vi "Telemetry Display.vi"() -> ()   [LabVIEW 2015]
uses:
  FPGA Telemetry.ctl
  Vehicle Status/Subsystem Status.ctl
  Vehicle Status/Subsystem Status Severity.ctl
  Vehicle Status/Subsystem Status Message.ctl
  AIR Status.ctl
  Reason for Shutdown.ctl
  Dash LED Status.ctl
  FPGA/SPI v2/ADXL345 Output.ctl
  CAN/MC/MC Telemetry.ctl
  CAN/MC/MC Temp 1.ctl
  CAN/MC/MC Temp 2.ctl
  CAN/MC/MC Temp 3.ctl
  CAN/MC/MC Current.ctl
  CAN/MC/MC Voltage.ctl
  CAN/MC/MC State.ctl
  CAN/Inverter States.ctl
  CAN/Inverter Run Modes.ctl
  CAN/VSM States.ctl
  CAN/MC/MC Torque.ctl
  CAN/MC/MC Position.ctl
  CAN/MC/MC Faults.ctl
  CAN/MC/MC Flux.ctl
  CAN/MC/MC Internal Voltages.ctl
  CAN/MC/MC Mod Index and Flux Weakening.ctl
  BMS Telemetry.ctl
  Session Information.ctl
  <vilib>/Math Plots/3D Math Plots/3D Bar/3D Bar XCtrl/3D Bar.xctl
  <vilib>/Math Plots/3D Math Plots/3D Bar/3D Bar Datatype/3D Bar Datatype.lvclass
  Vehicle Status/Remote Stop Type.ctl
  <vilib>/Math Plots/3D Math Plots/3D Bar/3D Bar Datatype/Public/Plot Helper (Matrix).vi
panel:
  out "Cell Temps":refnum<class "3D Plot Datatype.lvclass">[](xcontrol)
  out "Cell Voltages":refnum<class "3D Plot Datatype.lvclass">[](xcontrol)
  out "Waveform Chart":dbl(graph)=1.6
  out "Session Information":T1={"CLogFilePrefix"="110616 214028", "CExtraNotes"="", "CCircuit"="", "CCarName"="", "CDriverName"="", "CSessionDescription"=""}
  in  "Transmit":bool=TRUE
  in  "New TDMS Files":bool
  out "BMS Telemetry":T2={"bBMSIgnition"=FALSE, "bBMSChargerMains"=FALSE, "bBMSFastCharge"=FALSE, "bBMSChargerEnabled"=FALSE, "eBMSCarState"=enum."Off", "eBMSChargingState"=enum."Main Charging", "tBMSChargeStage"=12, "eBMSLastChargeError"=enum."No Error", "NBMSNumCells"=70, "bBMSUnderVProtection"=FALSE, "bBMSOverVProtection"=FALSE, "bBMSOverTProtection"=FALSE, "bBMSLeakageProtection"=FALSE, "bBMSNoCellCommsError"=FALSE, "bBMSLowVReduction"=FALSE, "bBMSHighTReduction"=FALSE, "VCellMin"=3.87, "VCellMax"=3.92, "VCellMean"=3.9, "VTotal"=273.18, "TCellMin"=29.0, "TCellMax"=42.0, "TCellMean"=32.0, "VCells"={"[0]"=3.91, "[1]"=3.9, "[2]"=3.9, "[3]"=3.9, "[4]"=3.91, "[5]"=3.91, "[6]"=3.91, "[7]"=3.9, "[8]"=3.92, "[9]"=3.9, "[10]"=3.91, "[11]"=3.9, "[12]"=3.9, "[13]"=3.9, "[14]"=3.9, "[15]"=3.9, "[16]"=3.92, "[16] 2"=0.0, "[17]"=3.9, "[18]"=3.91, "[19]"=3.9, "[20]"=3.91, "[21]"=3.9, "[22]"=3.9, "[23]"=3.91, "[24]"=3.91, "[25]"=3.91, "[26]"=3.9, "[27]"=3.9, "[28]"=3.9, "[29]"=3.9, "[30]"=3.9, "[31]"=3.9, "[32]"=3.9, "[33]"=3.91, "[33] 2"=0.0, "[34]"=3.91, "[35]"=3.91, "[36]"=3.9, "[37]"=3.9, "[38]"=3.91, "[39]"=3.91, "[40]"=3.91, "[41]"=3.9, "[42]"=3.9, "[43]"=3.91, "[44]"=3.9, "[45]"=3.8899999999999997, "[46]"=3.91, "[47]"=3.9, "[48]"=3.9, "[49]"=3.9, "[50]"=3.9, "[50] 2"=0.0, "[51]"=3.91, "[52] 2"=3.91, "[54]"=3.9, "[53]"=3.9, "[55]"=3.9, "[56]"=3.9, "[57]"=3.91, "[58]"=3.9, "[59]"=3.9, "[60]"=3.9, "[61]"=3.91, "[62]"=3.87, "[63]"=3.9, "[64]"=3.9, "[65]"=3.9, "[66]"=3.9, "[67]"=3.91}, "TBMSCells"={"[55]"=32.0, "[56]"=32.0, "[57]"=32.0, "[58]"=34.0, "[59]"=33.0, "[60]"=34.0, "[61]"=33.0, "[62]"=32.0, "[63]"=36.0, "[64]"=36.0, "[65]"=32.0, "[66]"=33.0, "[67]"=34.0, "[68]"=32.0, "[69]"=30.0, "[70]"=31.0, "[17]"=30.0, "[38]"=30.0, "[39]"=29.0, "[40]"=30.0, "[41]"=29.0, "[42]"=30.0, "[43]"=31.0, "[44]"=30.0, "[45]"=30.0, "[46]"=30.0, "[47]"=31.0, "[48]"=30.0, "[49]"=32.0, "[50]"=32.0, "[51]"=31.0, "[52]"=32.0, "[53]"=32.0, "[54]"=32.0, "[21]"=32.0, "[22]"=32.0, "[23]"=32.0, "[24]"=34.0, "[25]"=32.0, "[26]"=34.0, "[27]"=36.0, "[28]"=36.0, "[29]"=32.0, "[30]"=32.0, "[31]"=32.0, "[32]"=32.0, "[33]"=30.0, "[34]"=31.0, "[35]"=33.0, "[36]"=33.0, "[37]"=31.0, "[0]"=32.0, "[1]"=31.0, "[2]"=31.0, "[3]"=31.0, "[4]"=32.0, "[5]"=42.0, "[6]"=42.0, "[7]"=32.0, "[8]"=36.0, "[9]"=32.0, "[10]"=38.0, "[11]"=33.0, "[12]"=37.0, "[13]"=34.0, "[14]"=34.0, "[15]"=33.0, "[16]"=37.0}, "bChargerConnected"=TRUE, "VChargerSetpoint"=298.90000000000003, "IChargerSetpoint"=6.0, "VChargerActual"=277.7, "IChargerActual"=4.800000000000001, "BCells"={"[51]"=0.0, "[52]"=0.0, "[53]"=0.0, "[54]"=0.0, "[55]"=0.0, "[56]"=0.0, "[57]"=0.7843137254901961, "[58]"=0.0, "[59]"=1.5686274509803921, "[60]"=1.5686274509803921, "[61]"=0.0, "[62]"=0.0, "[63]"=0.7843137254901961, "[64]"=0.0, "[65]"=0.0, "[66]"=0.0, "[67]"=0.39215686274509803, "[34]"=0.39215686274509803, "[35]"=0.0, "[36]"=0.0, "[37]"=0.0, "[38]"=0.0, "[39]"=0.7843137254901961, "[40]"=0.0, "[41]"=0.0, "[42]"=0.0, "[43]"=8.627450980392156, "[44]"=0.0, "[45]"=0.0, "[46]"=0.7843137254901961, "[47]"=0.0, "[48]"=0.0, "[49]"=0.0, "[50]"=0.0, "[17]"=0.0, "[18]"=2.3529411764705883, "[19]"=0.0, "[20]"=0.0, "[21]"=0.0, "[22]"=0.0, "[23]"=1.5686274509803921, "[24]"=1.5686274509803921, "[25]"=0.0, "[26]"=0.0, "[27]"=0.0, "[28]"=0.0, "[29]"=0.0, "[30]"=0.0, "[31]"=0.0, "[32]"=0.0, "[33]"=0.0, "[0]"=0.0, "[1]"=0.0, "[2]"=0.0, "[3]"=0.0, "[4]"=1.9607843137254901, "[5]"=32.15686274509804, "[6]"=32.15686274509804, "[7]"=0.0, "[8]"=1.5686274509803921, "[9]"=0.0, "[10]"=16.07843137254902, "[11]"=0.0, "[12]"=3.9215686274509802, "[13]"=0.0, "[14]"=0.0, "[15]"=0.0, "[16]"=0.7843137254901961}, "bNewVCellMinSample"=TRUE, "Battery Temp"={"[0]"=0.0, "[1]"=0.0, "[2]"=0.0, "[3]"=0.0, "[4]"=0.0, "[5]"=0.0, "[6]"=0.0, "[7]"=0.0, "[8]"=0.0, "[9]"=0.0, "[10]"=0.0, "[11]"=0.0, "[12]"=0.0, "[13]"=0.0, "[14]"=0.0, "[15]"=0.0, "[16]"=0.0, "[17]"=0.0, "[18]"=0.0, "[19]"=0.0, "[20]"=0.0, "[21]"=0.0, "[22]"=0.0, "[23]"=0.0, "[24]"=0.0, "[25]"=0.0, "[26]"=0.0, "[27]"=0.0, "[28]"=0.0, "[29]"=0.0, "[30]"=0.0, "[31]"=0.0, "[32]"=0.0, "[33]"=0.0, "[34]"=0.0, "[35]"=0.0, "[36]"=0.0, "[37]"=0.0, "[38]"=0.0, "[39]"=0.0, "[40]"=0.0, "[41]"=0.0, "[42]"=0.0, "[43]"=0.0, "[44]"=0.0, "[45]"=0.0, "[46]"=0.0, "[47]"=0.0, "[48]"=0.0, "[49]"=0.0, "[50]"=0.0, "[51]"=0.0, "[52]"=0.0, "[53]"=0.0, "[54]"=0.0, "[55]"=0.0, "[56]"=0.0, "[57]"=0.0, "[58]"=0.0, "[59]"=0.0, "[60]"=0.0, "[61]"=0.0, "[62]"=0.0, "[63]"=0.0, "[64]"=0.0, "[65]"=0.0, "[66]"=0.0, "[67]"=0.0, "[68]"=0.0, "[69]"=0.0, "[71]"=0.0, "[70]"=0.0, "[0] 2"=0.0, "[1] 2"=0.0, "[2] 2"=0.0, "[3] 2"=0.0, "[4] 2"=0.0, "[5] 2"=0.0, "[6] 2"=0.0, "[7] 2"=0.0, "[8] 2"=0.0, "[9] 2"=0.0, "[10] 2"=0.0, "[11] 2"=0.0, "[12] 2"=0.0, "[13] 2"=0.0, "[14] 2"=0.0, "[15] 2"=0.0, "[16] 2"=0.0, "[17] 2"=0.0, "[18] 2"=0.0, "[19] 2"=0.0, "[20] 2"=0.0, "[21] 2"=0.0, "[22] 2"=0.0, "[23] 2"=0.0, "[24] 2"=0.0, "[25] 2"=0.0, "[26] 2"=0.0, "[27] 2"=0.0, "[28] 2"=0.0, "[29] 2"=0.0, "[30] 2"=0.0, "[31] 2"=0.0, "[32] 2"=0.0, "[33] 2"=0.0, "[34] 2"=0.0, "[35] 2"=0.0, "[36] 2"=0.0, "[37] 2"=0.0, "[38] 2"=0.0, "[39] 2"=0.0, "[40] 2"=0.0, "[41] 2"=0.0, "[42] 2"=0.0, "[43] 2"=0.0, "[44] 2"=0.0, "[45] 2"=0.0, "[46] 2"=0.0, "[47] 2"=0.0, "[48] 2"=0.0, "[49] 2"=0.0, "[50] 2"=0.0, "[51] 2"=0.0, "[52] 3"=0.0, "[53] 2"=0.0, "[54] 2"=0.0, "[55] 2"=0.0, "[56] 2"=0.0, "[57] 2"=0.0, "[58] 2"=0.0, "[59] 2"=0.0, "[60] 2"=0.0, "[61] 2"=0.0, "[62] 2"=0.0, "[63] 2"=0.0, "[64] 2"=0.0, "[65] 2"=0.0, "[66] 2"=0.0, "[67] 2"=0.0, "[68]2"=0.0, "[69]2"=0.0, "[70]2"=0.0, "[71]2"=0.0, "[0] 3"=0.0, "[1] 3"=0.0, "[2] 3"=0.0, "[3] 3"=0.0, "[4] 3"=0.0, "[5] 3"=0.0, "[6] 3"=0.0, "[7] 3"=0.0, "[8] 3"=0.0, "[9] 3"=0.0, "[10] 3"=0.0, "[11] 3"=0.0, "[12] 3"=0.0, "[13] 3"=0.0, "[14] 3"=0.0, "[15] 3"=0.0, "[16] 3"=0.0, "[17] 3"=0.0, "[18] 3"=0.0, "[19] 3"=0.0, "[20] 3"=0.0, "[21] 3"=0.0, "[22] 3"=0.0, "[23] 3"=0.0, "[24] 3"=0.0, "[25] 3"=0.0, "[26] 3"=0.0, "[27] 3"=0.0, "[28] 3"=0.0, "[29] 3"=0.0, "[30] 3"=0.0, "[31] 3"=0.0, "[32] 3"=0.0, "[33] 3"=0.0, "[34] 3"=0.0, "[35] 3"=0.0, "[36] 3"=0.0, "[37] 3"=0.0, "[38] 3"=0.0, "[39] 3"=0.0, "[40] 3"=0.0, "[41] 3"=0.0, "[42] 3"=0.0, "[43] 3"=0.0, "[44] 3"=0.0, "[45] 3"=0.0, "[46] 3"=0.0, "[47] 3"=0.0, "[48] 3"=0.0, "[49] 3"=0.0, "[50] 3"=0.0, "[51] 3"=0.0, "[52] 4"=0.0, "[53] 3"=0.0, "[54] 3"=0.0, "[55] 3"=0.0, "[56] 3"=0.0, "[57] 3"=0.0, "[58] 3"=0.0, "[59] 3"=0.0, "[60] 3"=0.0, "[61] 3"=0.0, "[62] 3"=0.0, "[63] 3"=0.0, "[64] 3"=0.0, "[65] 3"=0.0, "[66] 3"=0.0, "[67] 3"=0.0, "[68]3"=0.0, "[69]3"=0.0, "[70]3"=0.0, "[71]3"=0.0, "[4] 4"=0.0, "[5] 4"=0.0, "[6] 4"=0.0, "[7] 4"=0.0, "[8] 4"=0.0, "[9] 4"=0.0, "[10] 4"=0.0, "[11] 4"=0.0, "[12] 4"=0.0, "[13] 4"=0.0, "[14] 4"=0.0, "[15] 4"=0.0, "[16] 4"=0.0, "[17] 4"=0.0, "[18] 4"=0.0, "[19] 4"=0.0, "[20] 4"=0.0, "[21] 4"=0.0, "[22] 4"=0.0, "[23] 4"=0.0, "[24] 4"=0.0, "[25] 4"=0.0, "[26] 4"=0.0, "[27] 4"=0.0, "[28] 4"=0.0, "[29] 4"=0.0, "[30] 4"=0.0, "[31] 4"=0.0, "[32] 4"=0.0, "[33] 4"=0.0, "[17] 9"=0.0, "[0] 9"=0.0, "[51] 8"=0.0, "[34] 8"=0.0, "[17] 8"=0.0, "[0] 8"=0.0, "[34] 4"=0.0, "[35] 4"=0.0, "[36] 4"=0.0, "[37] 4"=0.0, "[38] 4"=0.0, "[39] 4"=0.0, "[40] 4"=0.0, "[41] 4"=0.0, "[42] 4"=0.0, "[43] 4"=0.0, "[44] 4"=0.0, "[45] 4"=0.0, "[46] 4"=0.0, "[47] 4"=0.0, "[48] 4"=0.0, "[49] 4"=0.0, "[50] 4"=0.0, "[34] 9"=0.0, "[51] 4"=0.0, "[52] 5"=0.0, "[53] 4"=0.0, "[54] 4"=0.0, "[55] 4"=0.0, "[56] 4"=0.0, "[57] 4"=0.0, "[58] 4"=0.0, "[59] 4"=0.0, "[60] 4"=0.0, "[61] 4"=0.0, "[62] 4"=0.0, "[63] 4"=0.0, "[64] 4"=0.0, "[65] 4"=0.0, "[66] 4"=0.0, "[67] 4"=0.0, "[51] 9"=0.0}, "TBMSMax"=0.0, "TBMSMin"=0.0, "TBMSMean"=0.0} {"TBMSMax" format="%#_13g"}
  in  "Return to Pits":bool
  in  "Remote Stop":bool
  in  "?":bool
  in  "Telem Stop":bool
  out "MC Telemetry":T3={"MC Temp 1"={"TMCModuleA"=32.0, "TMCModuleB"=32.3, "TMCModuleC"=31.9, "TMCGateDriver"=39.0}, "MC Temp 2"={"TMCControlBoard"=38.9, "TMCRTD1"=222.8, "TMCRTD2"=225.5, "TMCRTD3"=-1000.0}, "MC Temp 3"={"TMCRTD4"=-1000.0, "TMCRTD5"=-1000.0, "TMotor"=45.7, "MTorqueShudder"=0.0}, "MC Current"={"IMCPhaseA"=-0.8, "IMCPhaseB"=-0.8, "IMCPhaseC"=-1.2, "IMCBatteryCalc"=0.0}, "MC Voltage"={"VMCPhaseAB"=1.9, "VMCPhaseBC"=12.1, "VMCOutput"=0.0, "VMCBattery"=1.6}, "MC State"={"eMCInverterState"=enum."Idle Stop", "eMCInverterRunMode"=enum."Torque Mode", "eMCInverterCommandMode"=enum."CAN Mode", "bMCInverterEnable"=FALSE, "bMCInverterEnableLockout"=FALSE, "bMCDirectionForward"=FALSE, "eMCVSMState"=enum."VSM Wait", "bMCRelay1"=FALSE, "bMCRelay2"=FALSE, "bMCRelay3"=TRUE, "bMCRelay4"=FALSE}, "MC Torque"={"MMCRequested"=0.0, "MMCFeedback"=-0.5, "tMCElapsed"=0}, "MC Position"={"aMotor"=31.7, "nMotor"=0.0, "fMCOutput"=-0.1, "aDeltaResolverFilt"=112.2}, "MC Faults"={"MC Fault"={"Over-Speed"=FALSE, "Over-Current"=FALSE, "Over-Voltage"=FALSE, "Inverter Over-Temp"=FALSE, "Direction Command"=FALSE, "Inverter Response Time-Out"=FALSE, "Desat Fault"=FALSE, "Hardware Over-Current"=FALSE, "Under-Voltage"=FALSE, "CAN Command Message Lost"=FALSE, "Motor Over-Temp"=FALSE, "Module A Over-Temp"=FALSE, "Module B Over-Temp"=FALSE, "Module C Over-Temp"=FALSE, "PCB Over-Temp"=FALSE, "Gate Driver 1 Over-Temp"=FALSE, "Gate Driver 2 Over-Temp"=FALSE, "Gate Drive 3 Over-Temp"=FALSE, "Current Sensor Fault"=FALSE, "Resolver Not Connected"=FALSE}, "MC Post"=0, "MC RUN"=0}, "MC Flux"={"IMCFluxCommand"=0.0, "IMCFluxFeedback"=0.0, "IMC_Id"=0.0, "IMC_Iq"=0.0}, "MC Internal Voltages"={"VMCRef1_5"=0.0, "VMCRef2_5"=0.0, "VMCRef5"=0.0, "VMCRef12"=0.0}, "Mod Index & Flux Weakening"={"NMCModulationIndex"=0.0, "IMCFluxWeakeningOutput"=0.0, "IMCIdCommand"=0.0, "IMCIqCommand"=0.0}} {"MC Faults"."MC RUN" format="%x"; "MC Faults"."MC Post" format="%x"}
  out "Telemetry":T19={"CPU Load"={"Total (%)"=100.0, "Time Critical (%)"=0.7326315967249523, "Timed Structures (%)"=23.781649053291776, "High (%)"=8.916938850140745, "Above Normal (%)"=46.814152882047196, "Normal (%)"=19.754627617795332, "Background (%)"=0.0, "Idle (%)"=0.0, "ISR (%)"=0.0}, "SVehicleStatus"={"BMS Status"={"eStatusSeverity"=enum."Danger", "NValue"=42.0, "CMessage"=enum."BatteryTemperature", "bNotOK"=FALSE}, "MC Status"={"eStatusSeverity"=enum."Return to Pits", "NValue"=0.0, "CMessage"=enum."MCOverSpeed", "bNotOK"=FALSE}, "Shutdown Status"={"eStatusSeverity"=enum."Error", "NValue"=0.0, "CMessage"=enum."IMD", "bNotOK"=FALSE}, "sbRIO Status"={"eStatusSeverity"=enum."Return to Pits", "NValue"=59.75, "CMessage"=enum."sbRIOTemperature", "bNotOK"=FALSE}, "Vehicle Status"={"eStatusSeverity"=enum."Return to Pits", "NValue"=0.0, "CMessage"=enum."MCOverSpeed", "bNotOK"=FALSE}, "Shutdown State"=enum."Coolant Pump Started/AIR's On", "AIR Status"=enum."On", "Remote Return to Pits"=FALSE, "Reason for Shutdown"=enum."None", "MC State Machine Status"=enum."Disabled"}, "iPhone HF Data"={"gXiPhone"=0.0, "gYiPhone"=0.0, "gZiPhone"=0.0, "nYawXiPhone"=0.0, "nYawYiPhone"=0.0, "nYawZiPhone"=0.0}, "iPhone LF Data"={"nLatiPhone"=0.0, "nLongiPhone"=0.0, "nGPSiPhone"=0.0}, "stop"=TRUE, "VSupplyOffset"=8.890625, "VsbRIOSupply"=19.369203567504883, "bFPGALED"=TRUE, "TSBRIO"=60.0, "rTPS2Unscaled"=0.27203369140625, "rTPS1Unscaled"=0.0662841796875, "bTPSConsistent"=TRUE, "bTPSInRange"=TRUE, "rThrottle"=0.0029296875, "VTPS2"=1.2707386016845703, "rTPS2"=0.005859375, "VTPS1"=0.3103370666503906, "rTPS1"=0.0, "rTPS2Max"=0.155029296875, "rTPS2Min"=0.27294921875, "rTPS1Max"=0.179931640625, "rTPS1Min"=0.069091796875, "bCoolantPumpEnable"=FALSE, "bRTDSEnable"=FALSE, "bTSMSInStatus"=TRUE, "bPosAIREnable"=TRUE, "bBMSOK"=TRUE, "bIMDOK"=TRUE, "bBSPDOK"=TRUE, "bSBRIOOK2"=TRUE, "bSBRIOOK1"=TRUE, "bTSMSOutStatus"=TRUE, "eGreenDash"=enum."Off", "eYellowDash"=enum."Off", "eRedDash"=enum."Off", "bMotorControllerEnable"=FALSE, "tCurrentLap"=0, "bNewLap"=TRUE, "tLastLap"=1, "tLapMin"=0, "V5VSupply"=4.685937881469727, "bWheelRL"=FALSE, "bWheelRR"=FALSE, "bWheelFR"=FALSE, "bWheelFL"=FALSE, "VBrakePressureR"=0.4763374328613281, "VBrakePressureF"=0.46417808532714844, "bWheelRRStopped"=TRUE, "bWheelRLStopped"=TRUE, "bWheelFRStopped"=TRUE, "bWheelFLStopped"=TRUE, "tWheelRLPeriod"=0, "tWheelRRPeriod"=0, "tWheelFRPeriod"=0, "tWheelFLPeriod"=0, "bBrakeLight"=FALSE, "VShockRR"=-0.012302398681640625, "VShockRL"=-0.0151824951171875, "VShockFR"=-0.011661529541015625, "VShockFL"=-0.010061264038085938, "IHighCurrent"=-36.3125, "ILowCurrent"=-4.75, "pBrakeR"=7.95703125, "pBrakeF"=0.0, "bHighCurrentOK"=TRUE, "bLowCurrentOK"=TRUE, "bBrakeROK"=TRUE, "bBrakeFOK"=TRUE, "VSteerWheelMiddle"=2.5, "aSteerWheel"=156.627197265625, "nWheelFL"=0.0, "nWheelFR"=0.0, "nWheelRL"=0.0, "nWheelRR"=0.0, "ADXL345 Output"={"X"=0.0, "Y"=0.0, "Z"=0.0}, "Tire Diameter(m)"=0.529998779296875, "vWheelRR"=0.0, "vWheelRL"=0.0, "vWheelFR"=0.0, "vWheelFL"=0.0, "vWheelLowest"=0.0, "vWheelHighest"=0.0, "bAccel"=FALSE, "vAxleF"=0.0, "vCar"=0.0, "sLap"=0.0, "rSlipRL"=0.0, "rSlipRR"=0.0, "rSlipFL"=0.0, "rSlipFR"=0.0, "NLap"=221, "tLapReference"=0, "tFastestLap"=0, "MTorqueRequest"=0.0, "RS232 Error Out"={"status"=TRUE, "code"=-1073807252}} {"TSBRIO" format="%.10g"; "CPU Load"."ISR (%)" format="%#.2f"; "CPU Load"."Idle (%)" format="%#.2f"; "CPU Load"."Background (%)" format="%#.2f"; "CPU Load"."Normal (%)" format="%#.2f"; "CPU Load"."Above Normal (%)" format="%#.2f"; "CPU Load"."High (%)" format="%#.2g"; "CPU Load"."Time Critical (%)" format="%#.2g"}
  # "Inputs"
  # "Protection"
  # "State"
  # "Outputs"
  # "Reduction"
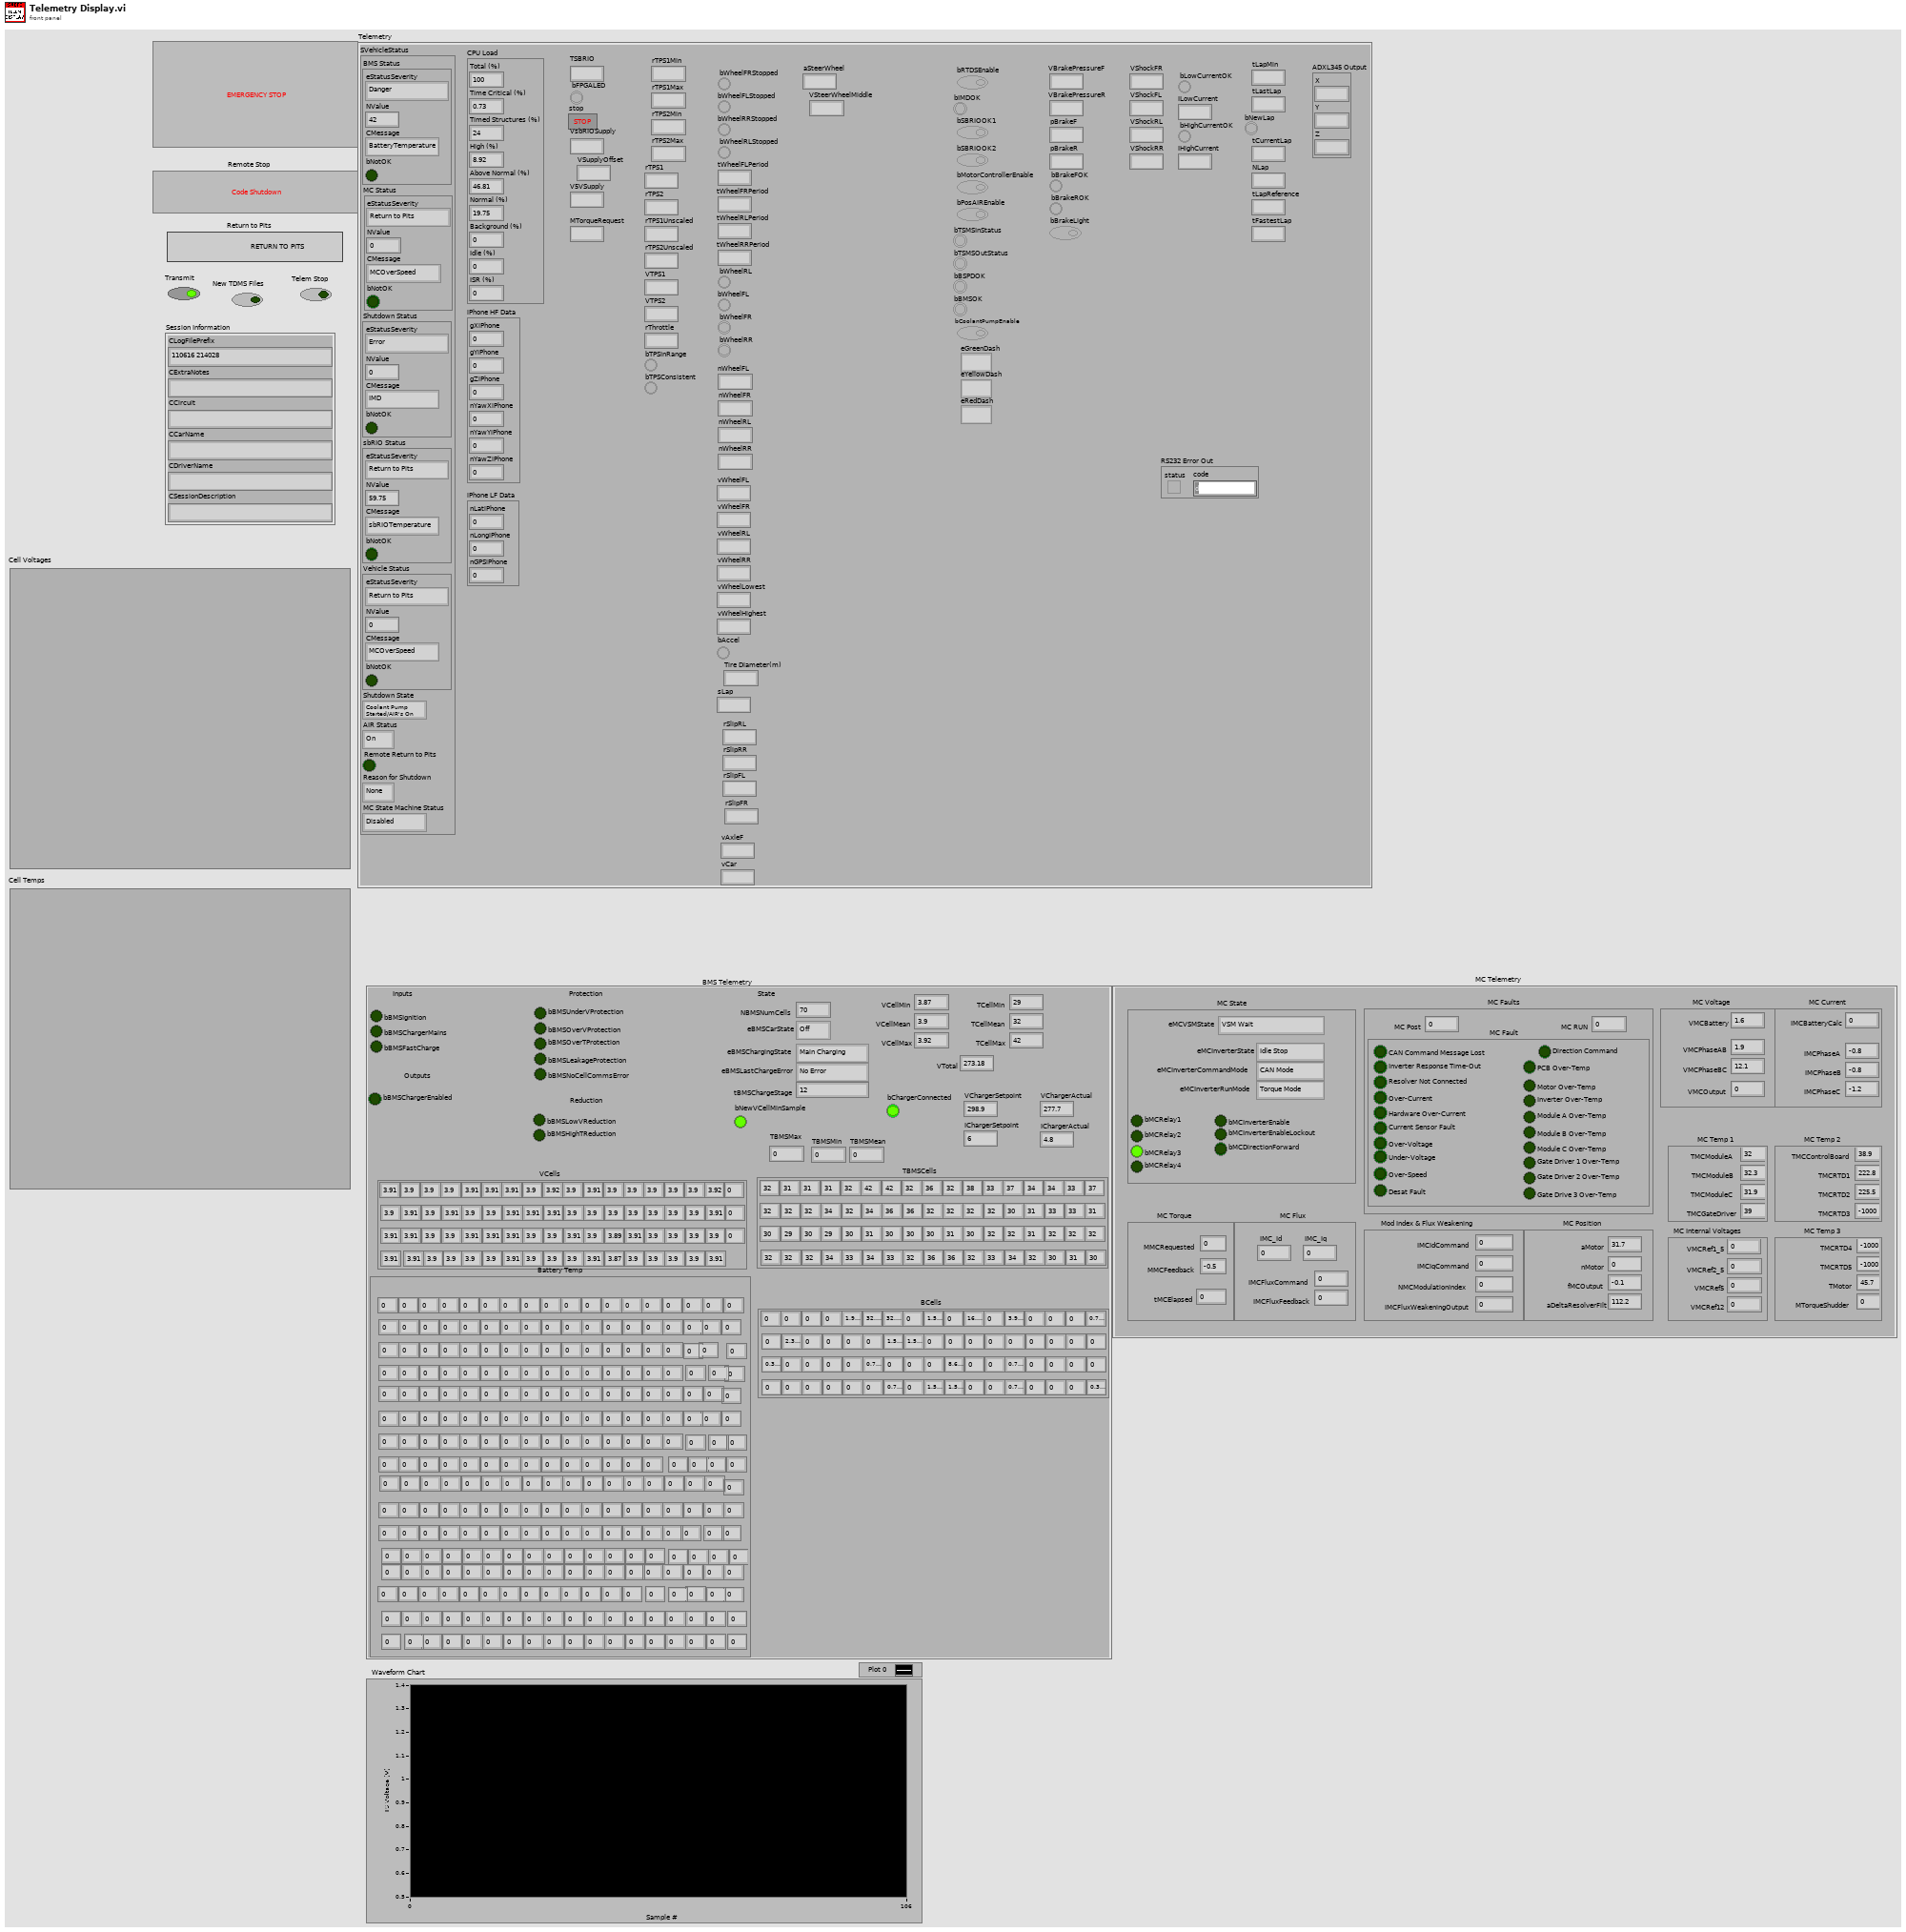
[diagram p1: front panel]
types:
  T1 = typedef "Session Information.ctl" = cluster{"CLogFilePrefix":string, "CExtraNotes":string, "CCircuit":string, "CCarName":string, "CDriverName":string, "CSessionDescription":string}
  T2 = typedef "BMS Telemetry.ctl" = cluster{"bBMSIgnition":bool, "bBMSChargerMains":bool, "bBMSFastCharge":bool, "bBMSChargerEnabled":bool, "eBMSCarState":enum16{"Off", "On, Not Charging", "Charging", "Charging Finished", "Charging Error"}, "eBMSChargingState":enum16{"Disconnected", "Pre-charging", "Main Charging", "Balancing", "Charging Finished OK", "Charging Error"}, "tBMSChargeStage":u16, "eBMSLastChargeError":enum16{"No Error", "No Cell Communication", "No Cell Communication - Non CAN Charger", "Maximum charging stage duration expired", "Cell Communication Lost during Charge", "Cannot set balancing voltage", "Cell temps too high", "No Comms so can't determine temp", "# of Cells Mismatch", "Cells Overvoltage", "Cell Protection Event occured."}, "NBMSNumCells":u8, "bBMSUnderVProtection":bool, "bBMSOverVProtection":bool, "bBMSOverTProtection":bool, "bBMSLeakageProtection":bool, "bBMSNoCellCommsError":bool, "bBMSLowVReduction":bool, "bBMSHighTReduction":bool, "VCellMin":dbl, "VCellMax":dbl, "VCellMean":dbl, "VTotal":dbl, "TCellMin":dbl, "TCellMax":dbl, "TCellMean":dbl, "VCells":cluster{"[0]":dbl, "[1]":dbl, "[2]":dbl, "[3]":dbl, "[4]":dbl, "[5]":dbl, "[6]":dbl, "[7]":dbl, "[8]":dbl, "[9]":dbl, "[10]":dbl, "[11]":dbl, "[12]":dbl, "[13]":dbl, "[14]":dbl, "[15]":dbl, "[16]":dbl, "[16] 2":dbl, "[17]":dbl, "[18]":dbl, "[19]":dbl, "[20]":dbl, "[21]":dbl, "[22]":dbl, "[23]":dbl, "[24]":dbl, "[25]":dbl, "[26]":dbl, "[27]":dbl, "[28]":dbl, "[29]":dbl, "[30]":dbl, "[31]":dbl, "[32]":dbl, "[33]":dbl, "[33] 2":dbl, "[34]":dbl, "[35]":dbl, "[36]":dbl, "[37]":dbl, "[38]":dbl, "[39]":dbl, "[40]":dbl, "[41]":dbl, "[42]":dbl, "[43]":dbl, "[44]":dbl, "[45]":dbl, "[46]":dbl, "[47]":dbl, "[48]":dbl, "[49]":dbl, "[50]":dbl, "[50] 2":dbl, "[51]":dbl, "[52] 2":dbl, "[54]":dbl, "[53]":dbl, "[55]":dbl, "[56]":dbl, "[57]":dbl, "[58]":dbl, "[59]":dbl, "[60]":dbl, "[61]":dbl, "[62]":dbl, "[63]":dbl, "[64]":dbl, "[65]":dbl, "[66]":dbl, "[67]":dbl}, "TBMSCells":cluster{"[55]":dbl, "[56]":dbl, "[57]":dbl, "[58]":dbl, "[59]":dbl, "[60]":dbl, "[61]":dbl, "[62]":dbl, "[63]":dbl, "[64]":dbl, "[65]":dbl, "[66]":dbl, "[67]":dbl, "[68]":dbl, "[69]":dbl, "[70]":dbl, "[17]":dbl, "[38]":dbl, "[39]":dbl, "[40]":dbl, "[41]":dbl, "[42]":dbl, "[43]":dbl, "[44]":dbl, "[45]":dbl, "[46]":dbl, "[47]":dbl, "[48]":dbl, "[49]":dbl, "[50]":dbl, "[51]":dbl, "[52]":dbl, "[53]":dbl, "[54]":dbl, "[21]":dbl, "[22]":dbl, "[23]":dbl, "[24]":dbl, "[25]":dbl, "[26]":dbl, "[27]":dbl, "[28]":dbl, "[29]":dbl, "[30]":dbl, "[31]":dbl, "[32]":dbl, "[33]":dbl, "[34]":dbl, "[35]":dbl, "[36]":dbl, "[37]":dbl, "[0]":dbl, "[1]":dbl, "[2]":dbl, "[3]":dbl, "[4]":dbl, "[5]":dbl, "[6]":dbl, "[7]":dbl, "[8]":dbl, "[9]":dbl, "[10]":dbl, "[11]":dbl, "[12]":dbl, "[13]":dbl, "[14]":dbl, "[15]":dbl, "[16]":dbl}, "bChargerConnected":bool, "VChargerSetpoint":dbl, "IChargerSetpoint":dbl, "VChargerActual":dbl, "IChargerActual":dbl, "BCells":cluster{"[51]":dbl, "[52]":dbl, "[53]":dbl, "[54]":dbl, "[55]":dbl, "[56]":dbl, "[57]":dbl, "[58]":dbl, "[59]":dbl, "[60]":dbl, "[61]":dbl, "[62]":dbl, "[63]":dbl, "[64]":dbl, "[65]":dbl, "[66]":dbl, "[67]":dbl, "[34]":dbl, "[35]":dbl, "[36]":dbl, "[37]":dbl, "[38]":dbl, "[39]":dbl, "[40]":dbl, "[41]":dbl, "[42]":dbl, "[43]":dbl, "[44]":dbl, "[45]":dbl, "[46]":dbl, "[47]":dbl, "[48]":dbl, "[49]":dbl, "[50]":dbl, "[17]":dbl, "[18]":dbl, "[19]":dbl, "[20]":dbl, "[21]":dbl, "[22]":dbl, "[23]":dbl, "[24]":dbl, "[25]":dbl, "[26]":dbl, "[27]":dbl, "[28]":dbl, "[29]":dbl, "[30]":dbl, "[31]":dbl, "[32]":dbl, "[33]":dbl, "[0]":dbl, "[1]":dbl, "[2]":dbl, "[3]":dbl, "[4]":dbl, "[5]":dbl, "[6]":dbl, "[7]":dbl, "[8]":dbl, "[9]":dbl, "[10]":dbl, "[11]":dbl, "[12]":dbl, "[13]":dbl, "[14]":dbl, "[15]":dbl, "[16]":dbl}, "bNewVCellMinSample":bool, "Battery Temp":cluster{"[0]":dbl, "[1]":dbl, "[2]":dbl, "[3]":dbl, "[4]":dbl, "[5]":dbl, "[6]":dbl, "[7]":dbl, "[8]":dbl, "[9]":dbl, "[10]":dbl, "[11]":dbl, "[12]":dbl, "[13]":dbl, "[14]":dbl, "[15]":dbl, "[16]":dbl, "[17]":dbl, "[18]":dbl, "[19]":dbl, "[20]":dbl, "[21]":dbl, "[22]":dbl, "[23]":dbl, "[24]":dbl, "[25]":dbl, "[26]":dbl, "[27]":dbl, "[28]":dbl, "[29]":dbl, "[30]":dbl, "[31]":dbl, "[32]":dbl, "[33]":dbl, "[34]":dbl, "[35]":dbl, "[36]":dbl, "[37]":dbl, "[38]":dbl, "[39]":dbl, "[40]":dbl, "[41]":dbl, "[42]":dbl, "[43]":dbl, "[44]":dbl, "[45]":dbl, "[46]":dbl, "[47]":dbl, "[48]":dbl, "[49]":dbl, "[50]":dbl, "[51]":dbl, "[52]":dbl, "[53]":dbl, "[54]":dbl, "[55]":dbl, "[56]":dbl, "[57]":dbl, "[58]":dbl, "[59]":dbl, "[60]":dbl, "[61]":dbl, "[62]":dbl, "[63]":dbl, "[64]":dbl, "[65]":dbl, "[66]":dbl, "[67]":dbl, "[68]":dbl, "[69]":dbl, "[71]":dbl, "[70]":dbl, "[0] 2":dbl, "[1] 2":dbl, "[2] 2":dbl, "[3] 2":dbl, "[4] 2":dbl, "[5] 2":dbl, "[6] 2":dbl, "[7] 2":dbl, "[8] 2":dbl, "[9] 2":dbl, "[10] 2":dbl, "[11] 2":dbl, "[12] 2":dbl, "[13] 2":dbl, "[14] 2":dbl, "[15] 2":dbl, "[16] 2":dbl, "[17] 2":dbl, "[18] 2":dbl, "[19] 2":dbl, "[20] 2":dbl, "[21] 2":dbl, "[22] 2":dbl, "[23] 2":dbl, "[24] 2":dbl, "[25] 2":dbl, "[26] 2":dbl, "[27] 2":dbl, "[28] 2":dbl, "[29] 2":dbl, "[30] 2":dbl, "[31] 2":dbl, "[32] 2":dbl, "[33] 2":dbl, "[34] 2":dbl, "[35] 2":dbl, "[36] 2":dbl, "[37] 2":dbl, "[38] 2":dbl, "[39] 2":dbl, "[40] 2":dbl, "[41] 2":dbl, "[42] 2":dbl, "[43] 2":dbl, "[44] 2":dbl, "[45] 2":dbl, "[46] 2":dbl, "[47] 2":dbl, "[48] 2":dbl, "[49] 2":dbl, "[50] 2":dbl, "[51] 2":dbl, "[52] 3":dbl, "[53] 2":dbl, "[54] 2":dbl, "[55] 2":dbl, "[56] 2":dbl, "[57] 2":dbl, "[58] 2":dbl, "[59] 2":dbl, "[60] 2":dbl, "[61] 2":dbl, "[62] 2":dbl, "[63] 2":dbl, "[64] 2":dbl, "[65] 2":dbl, "[66] 2":dbl, "[67] 2":dbl, "[68]2":dbl, "[69]2":dbl, "[70]2":dbl, "[71]2":dbl, "[0] 3":dbl, "[1] 3":dbl, "[2] 3":dbl, "[3] 3":dbl, "[4] 3":dbl, "[5] 3":dbl, "[6] 3":dbl, "[7] 3":dbl, "[8] 3":dbl, "[9] 3":dbl, "[10] 3":dbl, "[11] 3":dbl, "[12] 3":dbl, "[13] 3":dbl, "[14] 3":dbl, "[15] 3":dbl, "[16] 3":dbl, "[17] 3":dbl, "[18] 3":dbl, "[19] 3":dbl, "[20] 3":dbl, "[21] 3":dbl, "[22] 3":dbl, "[23] 3":dbl, "[24] 3":dbl, "[25] 3":dbl, "[26] 3":dbl, "[27] 3":dbl, "[28] 3":dbl, "[29] 3":dbl, "[30] 3":dbl, "[31] 3":dbl, "[32] 3":dbl, "[33] 3":dbl, "[34] 3":dbl, "[35] 3":dbl, "[36] 3":dbl, "[37] 3":dbl, "[38] 3":dbl, "[39] 3":dbl, "[40] 3":dbl, "[41] 3":dbl, "[42] 3":dbl, "[43] 3":dbl, "[44] 3":dbl, "[45] 3":dbl, "[46] 3":dbl, "[47] 3":dbl, "[48] 3":dbl, "[49] 3":dbl, "[50] 3":dbl, "[51] 3":dbl, "[52] 4":dbl, "[53] 3":dbl, "[54] 3":dbl, "[55] 3":dbl, "[56] 3":dbl, "[57] 3":dbl, "[58] 3":dbl, "[59] 3":dbl, "[60] 3":dbl, "[61] 3":dbl, "[62] 3":dbl, "[63] 3":dbl, "[64] 3":dbl, "[65] 3":dbl, "[66] 3":dbl, "[67] 3":dbl, "[68]3":dbl, "[69]3":dbl, "[70]3":dbl, "[71]3":dbl, "[4] 4":dbl, "[5] 4":dbl, "[6] 4":dbl, "[7] 4":dbl, "[8] 4":dbl, "[9] 4":dbl, "[10] 4":dbl, "[11] 4":dbl, "[12] 4":dbl, "[13] 4":dbl, "[14] 4":dbl, "[15] 4":dbl, "[16] 4":dbl, "[17] 4":dbl, "[18] 4":dbl, "[19] 4":dbl, "[20] 4":dbl, "[21] 4":dbl, "[22] 4":dbl, "[23] 4":dbl, "[24] 4":dbl, "[25] 4":dbl, "[26] 4":dbl, "[27] 4":dbl, "[28] 4":dbl, "[29] 4":dbl, "[30] 4":dbl, "[31] 4":dbl, "[32] 4":dbl, "[33] 4":dbl, "[17] 9":dbl, "[0] 9":dbl, "[51] 8":dbl, "[34] 8":dbl, "[17] 8":dbl, "[0] 8":dbl, "[34] 4":dbl, "[35] 4":dbl, "[36] 4":dbl, "[37] 4":dbl, "[38] 4":dbl, "[39] 4":dbl, "[40] 4":dbl, "[41] 4":dbl, "[42] 4":dbl, "[43] 4":dbl, "[44] 4":dbl, "[45] 4":dbl, "[46] 4":dbl, "[47] 4":dbl, "[48] 4":dbl, "[49] 4":dbl, "[50] 4":dbl, "[34] 9":dbl, "[51] 4":dbl, "[52] 5":dbl, "[53] 4":dbl, "[54] 4":dbl, "[55] 4":dbl, "[56] 4":dbl, "[57] 4":dbl, "[58] 4":dbl, "[59] 4":dbl, "[60] 4":dbl, "[61] 4":dbl, "[62] 4":dbl, "[63] 4":dbl, "[64] 4":dbl, "[65] 4":dbl, "[66] 4":dbl, "[67] 4":dbl, "[51] 9":dbl}, "TBMSMax":dbl, "TBMSMin":dbl, "TBMSMean":dbl}
  T3 = typedef "MC Telemetry.ctl" = cluster{"MC Temp 1":T4, "MC Temp 2":T5, "MC Temp 3":T6, "MC Current":T7, "MC Voltage":T8, "MC State":T9, "MC Torque":T13, "MC Position":T14, "MC Faults":T15, "MC Flux":T16, "MC Internal Voltages":T17, "Mod Index & Flux Weakening":T18}
  T4 = typedef "MC Temp 1.ctl" = cluster{"TMCModuleA":dbl, "TMCModuleB":dbl, "TMCModuleC":dbl, "TMCGateDriver":dbl}
  T5 = typedef "MC Temp 2.ctl" = cluster{"TMCControlBoard":dbl, "TMCRTD1":dbl, "TMCRTD2":dbl, "TMCRTD3":dbl}
  T6 = typedef "MC Temp 3.ctl" = cluster{"TMCRTD4":dbl, "TMCRTD5":dbl, "TMotor":dbl, "MTorqueShudder":dbl}
  T7 = typedef "MC Current.ctl" = cluster{"IMCPhaseA":dbl, "IMCPhaseB":dbl, "IMCPhaseC":dbl, "IMCBatteryCalc":dbl}
  T8 = typedef "MC Voltage.ctl" = cluster{"VMCPhaseAB":dbl, "VMCPhaseBC":dbl, "VMCOutput":dbl, "VMCBattery":dbl}
  T9 = typedef "MC State.ctl" = cluster{"eMCInverterState":T10, "eMCInverterRunMode":T11, "eMCInverterCommandMode":enum16{"CAN Mode", "VSM Mode"}, "bMCInverterEnable":bool, "bMCInverterEnableLockout":bool, "bMCDirectionForward":bool, "eMCVSMState":T12, "bMCRelay1":bool, "bMCRelay2":bool, "bMCRelay3":bool, "bMCRelay4":bool}
  T10 = typedef "Inverter States.ctl" = enum16{"Power On", "Stop", "Open Loop", "Closed Loop", "Wait", "Internal", "Idle Run", "Idle Stop", ""}
  T11 = typedef "Inverter Run Modes.ctl" = enum16{"Torque Mode", "Speed Mode"}
  T12 = typedef "VSM States.ctl" = enum16{"VSM Start", "Pre-Charge Init", "Pre-Charge Active", "Pre-Charge Complete", "VSM Wait", "VSM Ready", "Motor Running", "Blink Fault Code", "Shutdown in Process", "Recycle Power"}
  T13 = typedef "MC Torque.ctl" = cluster{"MMCRequested":dbl, "MMCFeedback":dbl, "tMCElapsed":u32}
  T14 = typedef "MC Position.ctl" = cluster{"aMotor":dbl, "nMotor":dbl, "fMCOutput":dbl, "aDeltaResolverFilt":dbl}
  T15 = typedef "MC Faults.ctl" = cluster{"MC Fault":cluster{"Over-Speed":bool, "Over-Current":bool, "Over-Voltage":bool, "Inverter Over-Temp":bool, "Direction Command":bool, "Inverter Response Time-Out":bool, "Desat Fault":bool, "Hardware Over-Current":bool, "Under-Voltage":bool, "CAN Command Message Lost":bool, "Motor Over-Temp":bool, "Module A Over-Temp":bool, "Module B Over-Temp":bool, "Module C Over-Temp":bool, "PCB Over-Temp":bool, "Gate Driver 1 Over-Temp":bool, "Gate Driver 2 Over-Temp":bool, "Gate Drive 3 Over-Temp":bool, "Current Sensor Fault":bool, "Resolver Not Connected":bool}, "MC Post":u32, "MC RUN":u32}
  T16 = typedef "MC Flux.ctl" = cluster{"IMCFluxCommand":dbl, "IMCFluxFeedback":dbl, "IMC_Id":dbl, "IMC_Iq":dbl}
  T17 = typedef "MC Internal Voltages.ctl" = cluster{"VMCRef1_5":dbl, "VMCRef2_5":dbl, "VMCRef5":dbl, "VMCRef12":dbl}
  T18 = typedef "MC Mod Index and Flux Weakening.ctl" = cluster{"NMCModulationIndex":dbl, "IMCFluxWeakeningOutput":dbl, "IMCIdCommand":dbl, "IMCIqCommand":dbl}
  T19 = typedef "FPGA Telemetry.ctl" = cluster{"CPU Load":cluster{"Total (%)":dbl, "Time Critical (%)":dbl, "Timed Structures (%)":dbl, "High (%)":dbl, "Above Normal (%)":dbl, "Normal (%)":dbl, "Background (%)":dbl, "Idle (%)":dbl, "ISR (%)":dbl}, "SVehicleStatus":cluster{"BMS Status":T20, "MC Status":T20, "Shutdown Status":T20, "sbRIO Status":T20, "Vehicle Status":T20, "Shutdown State":enum16{"NI.SC.Initial", "NI.SC.History", "NI.SC.ShallowHistory", "NI.SC.Terminal", "Coolant Pump Started/AIR's On", "AIRs On", "Precharge", "TSMS Off"}, "AIR Status":T23, "Remote Return to Pits":bool, "Reason for Shutdown":T24, "MC State Machine Status":enum16{"NI.SC.Initial", "NI.SC.History", "NI.SC.ShallowHistory", "NI.SC.Terminal", "Broadcast Diag", "Let Current Drop then Disable AIR's", "Enabled", "Disabled"}}, "iPhone HF Data":cluster{"gXiPhone":dbl, "gYiPhone":dbl, "gZiPhone":dbl, "nYawXiPhone":dbl, "nYawYiPhone":dbl, "nYawZiPhone":dbl}, "iPhone LF Data":cluster{"nLatiPhone":dbl, "nLongiPhone":dbl, "nGPSiPhone":dbl}, "stop":bool, "VSupplyOffset":fxp<+,12,4>, "VsbRIOSupply":fxp<+/-,25,6>, "bFPGALED":bool, "TSBRIO":fxp<+/-,33,17>, "rTPS2Unscaled":fxp<+/-,16,1>, "rTPS1Unscaled":fxp<+/-,16,1>, "bTPSConsistent":bool, "bTPSInRange":bool, "rThrottle":fxp<+/-,33,22>, "VTPS2":fxp<+/-,24,5>, "rTPS2":fxp<+/-,31,22>, "VTPS1":fxp<+/-,24,5>, "rTPS1":fxp<+/-,31,22>, "rTPS2Max":fxp<+,16,4>, "rTPS2Min":fxp<+,16,4>, "rTPS1Max":fxp<+,16,4>, "rTPS1Min":fxp<+,16,4>, "bCoolantPumpEnable":bool, "bRTDSEnable":bool, "bTSMSInStatus":bool, "bPosAIREnable":bool, "bBMSOK":bool, "bIMDOK":bool, "bBSPDOK":bool, "bSBRIOOK2":bool, "bSBRIOOK1":bool, "bTSMSOutStatus":bool, "eGreenDash":T25, "eYellowDash":T25, "eRedDash":T25, "bMotorControllerEnable":bool, "tCurrentLap":u32, "bNewLap":bool, "tLastLap":u32, "tLapMin":u32, "V5VSupply":fxp<+/-,24,5>, "bWheelRL":bool, "bWheelRR":bool, "bWheelFR":bool, "bWheelFL":bool, "VBrakePressureR":fxp<+/-,24,5>, "VBrakePressureF":fxp<+/-,24,5>, "bWheelRRStopped":bool, "bWheelRLStopped":bool, "bWheelFRStopped":bool, "bWheelFLStopped":bool, "tWheelRLPeriod":u32, "tWheelRRPeriod":u32, "tWheelFRPeriod":u32, "tWheelFLPeriod":u32, "bBrakeLight":bool, "VShockRR":fxp<+/-,24,5>, "VShockRL":fxp<+/-,24,5>, "VShockFR":fxp<+/-,24,5>, "VShockFL":fxp<+/-,24,5>, "IHighCurrent":fxp<+/-,24,15>, "ILowCurrent":fxp<+/-,24,15>, "pBrakeR":fxp<+,26,13>, "pBrakeF":fxp<+,26,13>, "bHighCurrentOK":bool, "bLowCurrentOK":bool, "bBrakeROK":bool, "bBrakeFOK":bool, "VSteerWheelMiddle":fxp<+/-,26,5>, "aSteerWheel":fxp<+/-,31,13>, "nWheelFL":fxp<+/-,32,16>, "nWheelFR":fxp<+/-,32,16>, "nWheelRL":fxp<+/-,32,16>, "nWheelRR":fxp<+/-,32,16>, "ADXL345 Output":T26, "Tire Diameter(m)":fxp<+,16,1>, "vWheelRR":fxp<+/-,32,18>, "vWheelRL":fxp<+/-,32,18>, "vWheelFR":fxp<+/-,32,18>, "vWheelFL":fxp<+/-,32,18>, "vWheelLowest":fxp<+/-,32,18>, "vWheelHighest":fxp<+/-,32,18>, "bAccel":bool, "vAxleF":fxp<+/-,33,19>, "vCar":fxp<+/-,33,19>, "sLap":fxp<+,32,12>, "rSlipRL":fxp<+/-,12,1>, "rSlipRR":fxp<+/-,12,1>, "rSlipFL":fxp<+/-,12,1>, "rSlipFR":fxp<+/-,12,1>, "NLap":u8, "tLapReference":u32, "tFastestLap":u32, "MTorqueRequest":dbl, "RS232 Error Out":cluster{"status":bool, "code":i32}}
  T20 = typedef "Subsystem Status.ctl" = cluster{"eStatusSeverity":T21, "NValue":sgl, "CMessage":T22, "bNotOK":bool}
  T21 = typedef "Subsystem Status Severity.ctl" = enum16{"Okay", "Short Warning", "Long Warning", "Return to Pits", "Error", "Danger"}
  T22 = typedef "Subsystem Status Message.ctl" = enum16{"ControllerTemperature", "MotorTemperature", "BatteryTemperature", "BatteryLowVoltage", "LVBattery", "sbRIOTemperature", "Precharge", "BSPD", "IMD", "RemoteReturnToPits", "EStopInterrupted", "NoCellComms", "MCOverSpeed", "MCOverCurrent", "MCOverVoltage", "MCInverterOverTemp", "MCDirectionCommand", "MCInverterTimeout", "MCDesatFault", "MCHWOverCurrent", "MCUnderVoltage", "MCCommandMessageLost", "MotorOverTemp", "MCModAOverTemp", "MCModBOverTemp", "MCModCOverTemp", "MCPCBOverTemp", "MCGateDrv1OverTemp", "MCDateDrv2OverTemp", "MCCurrentSensorFault", "MCResolverNotConnected", "ShutdownLatchTripped", "UnknownBMS", "RemoteEmergency"}
  T23 = typedef "AIR Status.ctl" = enum16{"Off", "Precharge", "On"}
  T24 = typedef "Reason for Shutdown.ctl" = enum16{"None", "BMS", "Shutdown", "sbRIO", "MC", "Remote"}
  T25 = typedef "Dash LED Status.ctl" = enum16{"Off", "Flashing", "On"}
  T26 = typedef "ADXL345 Output.ctl" = cluster{"X":fxp<+/-,14,4>, "Y":fxp<+/-,14,4>, "Z":fxp<+/-,14,4>}
  T27 = typedef "Remote Stop Type.ctl" = cluster{"bRemoteStop":bool, "bRemoteEmergencyStop":bool, "bRemoteReturnToPits":bool, "bRemoteNewLogs":bool}
  T28 = cluster{"[0]":dbl, "[1]":dbl, "[2]":dbl, "[3]":dbl, "[4]":dbl, "[5]":dbl, "[6]":dbl, "[7]":dbl, "[8]":dbl, "[9]":dbl, "[10]":dbl, "[11]":dbl, "[12]":dbl, "[13]":dbl, "[14]":dbl, "[15]":dbl, "[16]":dbl, "[16] 2":dbl, "[17]":dbl, "[18]":dbl, "[19]":dbl, "[20]":dbl, "[21]":dbl, "[22]":dbl, "[23]":dbl, "[24]":dbl, "[25]":dbl, "[26]":dbl, "[27]":dbl, "[28]":dbl, "[29]":dbl, "[30]":dbl, "[31]":dbl, "[32]":dbl, "[33]":dbl, "[33] 2":dbl, "[34]":dbl, "[35]":dbl, "[36]":dbl, "[37]":dbl, "[38]":dbl, "[39]":dbl, "[40]":dbl, "[41]":dbl, "[42]":dbl, "[43]":dbl, "[44]":dbl, "[45]":dbl, "[46]":dbl, "[47]":dbl, "[48]":dbl, "[49]":dbl, "[50]":dbl, "[50] 2":dbl, "[51]":dbl, "[52] 2":dbl, "[54]":dbl, "[53]":dbl, "[55]":dbl, "[56]":dbl, "[57]":dbl, "[58]":dbl, "[59]":dbl, "[60]":dbl, "[61]":dbl, "[62]":dbl, "[63]":dbl, "[64]":dbl, "[65]":dbl, "[66]":dbl, "[67]":dbl}
  T29 = cluster{"[55]":dbl, "[56]":dbl, "[57]":dbl, "[58]":dbl, "[59]":dbl, "[60]":dbl, "[61]":dbl, "[62]":dbl, "[63]":dbl, "[64]":dbl, "[65]":dbl, "[66]":dbl, "[67]":dbl, "[68]":dbl, "[69]":dbl, "[70]":dbl, "[17]":dbl, "[38]":dbl, "[39]":dbl, "[40]":dbl, "[41]":dbl, "[42]":dbl, "[43]":dbl, "[44]":dbl, "[45]":dbl, "[46]":dbl, "[47]":dbl, "[48]":dbl, "[49]":dbl, "[50]":dbl, "[51]":dbl, "[52]":dbl, "[53]":dbl, "[54]":dbl, "[21]":dbl, "[22]":dbl, "[23]":dbl, "[24]":dbl, "[25]":dbl, "[26]":dbl, "[27]":dbl, "[28]":dbl, "[29]":dbl, "[30]":dbl, "[31]":dbl, "[32]":dbl, "[33]":dbl, "[34]":dbl, "[35]":dbl, "[36]":dbl, "[37]":dbl, "[0]":dbl, "[1]":dbl, "[2]":dbl, "[3]":dbl, "[4]":dbl, "[5]":dbl, "[6]":dbl, "[7]":dbl, "[8]":dbl, "[9]":dbl, "[10]":dbl, "[11]":dbl, "[12]":dbl, "[13]":dbl, "[14]":dbl, "[15]":dbl, "[16]":dbl}
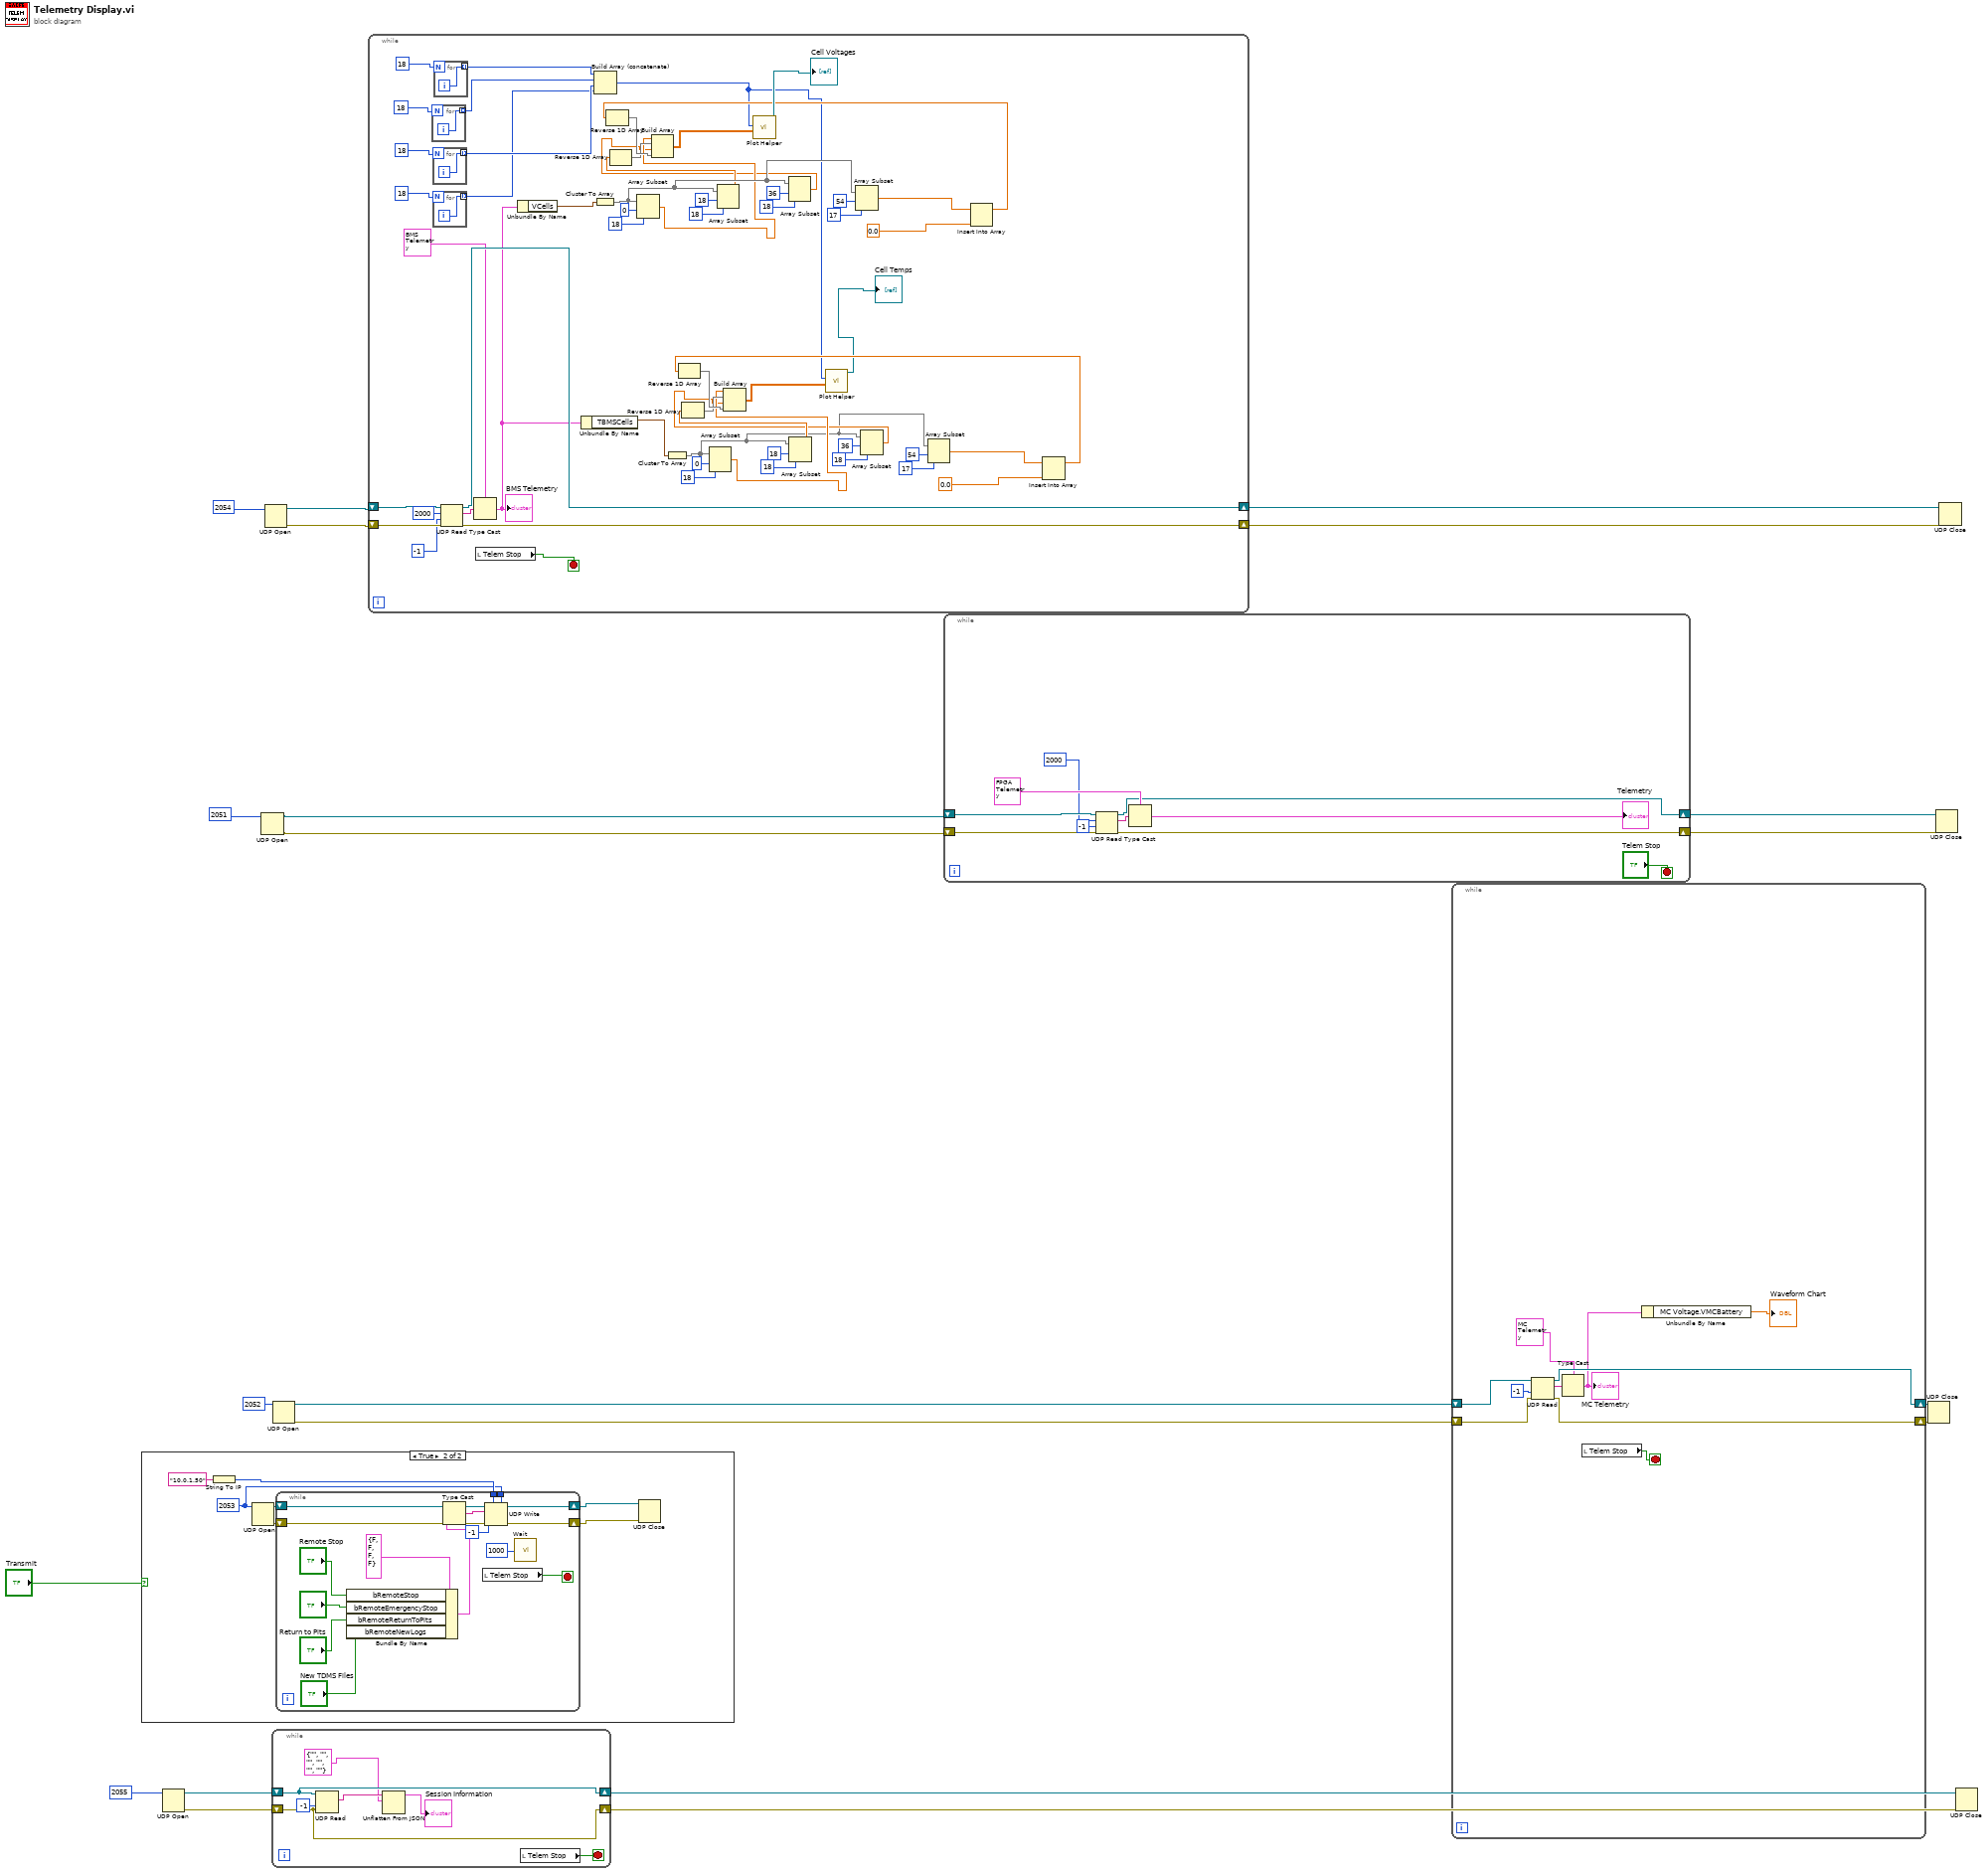
[diagram p0: block diagram]
diagram:
  n1 = case shown="True" "Transmit" {
    frame False {
    }
    frame True {
      w24 = u16 2053 ("port")
      n2 = String To IP(1:"10.0.1.50" ("name")) -> (0:w25:u32)
      n3 = UDP Open(11:w24) -> (port=w27:refnum<k16>, 0:w28:errorcluster)  [unwired: 4 in, 1 out]
      n4 = while {
        tunnel: w25 -> [w41]
        tunnel: w24 -> [w40]
        shift-right: [w39] -> w23
        shift-left: w27 -> [w42]
        shift-right: [w38] -> w22
        shift-left: w28 -> [w43]
        stop <- w36 stop-if-true
        n5 = Bundle By Name(cluster=T27 {"bRemoteStop"=FALSE, "bRemoteEmergencyStop"=FALSE, "bRemoteReturnToPits"=FALSE, "bRemoteNewLogs"=FALSE} ("Remote Signalling"), "bRemoteStop"="Remote Stop", "bRemoteEmergencyStop"="?", "bRemoteReturnToPits"="Return to Pits", "bRemoteNewLogs"="New TDMS Files") -> (w34:T27)
        n6 = Type Cast(x=w34) -> (*(type *) &x=w44:string)  [unwired: 1 in]
        n7 = local read "Telem Stop"() -> (w36:bool)
        n8 = UDP Write(address=w41, port or service name=w40, connection ID=w42, data in=w44, 8:w43, 9:-1 ("timeout ms (25000)")) -> (error out=w38:errorcluster, 3:w39:refnum<k16>)
        n9 = call "Wait"("Count(mSec)"=u32 1000) -> ()  [unwired: 1 out]
      }
      n10 = UDP Close(connection ID=w23, 8:w22) -> ()  [unwired: 2 out]
    }
  }
  n11 = UDP Open(11:u16 2055 ("port")) -> (port=w6:refnum<k16>, 0:w5:errorcluster)  [unwired: 4 in, 1 out]
  n12 = UDP Open(11:u16 2051 ("port")) -> (port=w13:refnum<k16>, 0:w12:errorcluster)  [unwired: 4 in, 1 out]
  n13 = UDP Open(11:u16 2054 ("port")) -> (port=w8:refnum<k16>, 0:w7:errorcluster)  [unwired: 4 in, 1 out]
  n14 = while {
    shift-right: [w49] -> w2
    shift-left: w6 -> [w49]
    shift-right: [w48] -> w3
    shift-left: w5 -> [w48]
    stop <- w50 stop-if-true
    n15 = UDP Read(connection ID=w49, timeout ms (25000)=-1, 8:w48) -> (data out=w51:string)  [unwired: 1 in, 4 out]
    n16 = Unflatten From JSON(JSON string=w51, type and defaults=T1 {"CLogFilePrefix"="", "CExtraNotes"="", "CCircuit"="", "CCarName"="", "CDriverName"="", "CSessionDescription"=""} ("Session Information")) -> (value=→"Session Information":T1)  [unwired: 5 in, 1 out]
    n17 = local read "Telem Stop"() -> (w50:bool)
  }
  n18 = UDP Open(11:u16 2052 ("port")) -> (port=w21:refnum<k16>, 0:w15:errorcluster)  [unwired: 4 in, 1 out]
  n19 = while {
    shift-right: [w107] -> w11
    shift-left: w7 -> [w108]
    shift-right: [w106] -> w10
    shift-left: w8 -> [w109]
    stop <- w105 stop-if-true
    n20 = for {
      N: 18 -> [_]
      tunnel: [w113] -> w94 mode=indexing
      i -> [w113]
    }
    n21 = for {
      N: 18 -> [_]
      tunnel: [w112] -> w93 mode=indexing
      i -> [w112]
    }
    n22 = for {
      N: 18 -> [_]
      tunnel: [w111] -> w92 mode=indexing
      i -> [w111]
    }
    n23 = for {
      N: 18 -> [_]
      tunnel: [w114] -> w95 mode=indexing
      i -> [w114]
    }
    n24 = UDP Read(connection ID=w109, max size (548)=2000, timeout ms (25000)=-1 ("max size (548)"), 8:w108) -> (data out=w110:string, error out=w107:errorcluster, 3:w106:refnum<k16>)  [unwired: 2 out]
    n25 = Type Cast(type=T2 {"bBMSIgnition"=FALSE, "bBMSChargerMains"=FALSE, "bBMSFastCharge"=FALSE, "bBMSChargerEnabled"=FALSE, "eBMSCarState"=enum."Off", "eBMSChargingState"=enum."Disconnected", "tBMSChargeStage"=0, "eBMSLastChargeError"=enum."No Error", "NBMSNumCells"=0, "bBMSUnderVProtection"=FALSE, "bBMSOverVProtection"=FALSE, "bBMSOverTProtection"=FALSE, "bBMSLeakageProtection"=FALSE, "bBMSNoCellCommsError"=FALSE, "bBMSLowVReduction"=FALSE, "bBMSHighTReduction"=FALSE, "VCellMin"=0.0, "VCellMax"=0.0, "VCellMean"=0.0, "VTotal"=0.0, "TCellMin"=0.0, "TCellMax"=0.0, "TCellMean"=0.0, "VCells"={"[0]"=0.0, "[1]"=0.0, "[2]"=0.0, "[3]"=0.0, "[4]"=0.0, "[5]"=0.0, "[6]"=0.0, "[7]"=0.0, "[8]"=0.0, "[9]"=0.0, "[10]"=0.0, "[11]"=0.0, "[12]"=0.0, "[13]"=0.0, "[14]"=0.0, "[15]"=0.0, "[16]"=0.0, "[16] 2"=0.0, "[17]"=0.0, "[18]"=0.0, "[19]"=0.0, "[20]"=0.0, "[21]"=0.0, "[22]"=0.0, "[23]"=0.0, "[24]"=0.0, "[25]"=0.0, "[26]"=0.0, "[27]"=0.0, "[28]"=0.0, "[29]"=0.0, "[30]"=0.0, "[31]"=0.0, "[32]"=0.0, "[33]"=0.0, "[33] 2"=0.0, "[34]"=0.0, "[35]"=0.0, "[36]"=0.0, "[37]"=0.0, "[38]"=0.0, "[39]"=0.0, "[40]"=0.0, "[41]"=0.0, "[42]"=0.0, "[43]"=0.0, "[44]"=0.0, "[45]"=0.0, "[46]"=0.0, "[47]"=0.0, "[48]"=0.0, "[49]"=0.0, "[50]"=0.0, "[50] 2"=0.0, "[51]"=0.0, "[52] 2"=0.0, "[54]"=0.0, "[53]"=0.0, "[55]"=0.0, "[56]"=0.0, "[57]"=0.0, "[58]"=0.0, "[59]"=0.0, "[60]"=0.0, "[61]"=0.0, "[62]"=0.0, "[63]"=0.0, "[64]"=0.0, "[65]"=0.0, "[66]"=0.0, "[67]"=0.0}, "TBMSCells"={"[55]"=0.0, "[56]"=0.0, "[57]"=0.0, "[58]"=0.0, "[59]"=0.0, "[60]"=0.0, "[61]"=0.0, "[62]"=0.0, "[63]"=0.0, "[64]"=0.0, "[65]"=0.0, "[66]"=0.0, "[67]"=0.0, "[68]"=0.0, "[69]"=0.0, "[70]"=0.0, "[17]"=0.0, "[38]"=0.0, "[39]"=0.0, "[40]"=0.0, "[41]"=0.0, "[42]"=0.0, "[43]"=0.0, "[44]"=0.0, "[45]"=0.0, "[46]"=0.0, "[47]"=0.0, "[48]"=0.0, "[49]"=0.0, "[50]"=0.0, "[51]"=0.0, "[52]"=0.0, "[53]"=0.0, "[54]"=0.0, "[21]"=0.0, "[22]"=0.0, "[23]"=0.0, "[24]"=0.0, "[25]"=0.0, "[26]"=0.0, "[27]"=0.0, "[28]"=0.0, "[29]"=0.0, "[30]"=0.0, "[31]"=0.0, "[32]"=0.0, "[33]"=0.0, "[34]"=0.0, "[35]"=0.0, "[36]"=0.0, "[37]"=0.0, "[0]"=0.0, "[1]"=0.0, "[2]"=0.0, "[3]"=0.0, "[4]"=0.0, "[5]"=0.0, "[6]"=0.0, "[7]"=0.0, "[8]"=0.0, "[9]"=0.0, "[10]"=0.0, "[11]"=0.0, "[12]"=0.0, "[13]"=0.0, "[14]"=0.0, "[15]"=0.0, "[16]"=0.0}, "bChargerConnected"=FALSE, "VChargerSetpoint"=0.0, "IChargerSetpoint"=0.0, "VChargerActual"=0.0, "IChargerActual"=0.0, "BCells"={"[51]"=0.0, "[52]"=0.0, "[53]"=0.0, "[54]"=0.0, "[55]"=0.0, "[56]"=0.0, "[57]"=0.0, "[58]"=0.0, "[59]"=0.0, "[60]"=0.0, "[61]"=0.0, "[62]"=0.0, "[63]"=0.0, "[64]"=0.0, "[65]"=0.0, "[66]"=0.0, "[67]"=0.0, "[34]"=0.0, "[35]"=0.0, "[36]"=0.0, "[37]"=0.0, "[38]"=0.0, "[39]"=0.0, "[40]"=0.0, "[41]"=0.0, "[42]"=0.0, "[43]"=0.0, "[44]"=0.0, "[45]"=0.0, "[46]"=0.0, "[47]"=0.0, "[48]"=0.0, "[49]"=0.0, "[50]"=0.0, "[17]"=0.0, "[18]"=0.0, "[19]"=0.0, "[20]"=0.0, "[21]"=0.0, "[22]"=0.0, "[23]"=0.0, "[24]"=0.0, "[25]"=0.0, "[26]"=0.0, "[27]"=0.0, "[28]"=0.0, "[29]"=0.0, "[30]"=0.0, "[31]"=0.0, "[32]"=0.0, "[33]"=0.0, "[0]"=0.0, "[1]"=0.0, "[2]"=0.0, "[3]"=0.0, "[4]"=0.0, "[5]"=0.0, "[6]"=0.0, "[7]"=0.0, "[8]"=0.0, "[9]"=0.0, "[10]"=0.0, "[11]"=0.0, "[12]"=0.0, "[13]"=0.0, "[14]"=0.0, "[15]"=0.0, "[16]"=0.0}, "bNewVCellMinSample"=FALSE, "Battery Temp"={"[0]"=0.0, "[1]"=0.0, "[2]"=0.0, "[3]"=0.0, "[4]"=0.0, "[5]"=0.0, "[6]"=0.0, "[7]"=0.0, "[8]"=0.0, "[9]"=0.0, "[10]"=0.0, "[11]"=0.0, "[12]"=0.0, "[13]"=0.0, "[14]"=0.0, "[15]"=0.0, "[16]"=0.0, "[17]"=0.0, "[18]"=0.0, "[19]"=0.0, "[20]"=0.0, "[21]"=0.0, "[22]"=0.0, "[23]"=0.0, "[24]"=0.0, "[25]"=0.0, "[26]"=0.0, "[27]"=0.0, "[28]"=0.0, "[29]"=0.0, "[30]"=0.0, "[31]"=0.0, "[32]"=0.0, "[33]"=0.0, "[34]"=0.0, "[35]"=0.0, "[36]"=0.0, "[37]"=0.0, "[38]"=0.0, "[39]"=0.0, "[40]"=0.0, "[41]"=0.0, "[42]"=0.0, "[43]"=0.0, "[44]"=0.0, "[45]"=0.0, "[46]"=0.0, "[47]"=0.0, "[48]"=0.0, "[49]"=0.0, "[50]"=0.0, "[51]"=0.0, "[52]"=0.0, "[53]"=0.0, "[54]"=0.0, "[55]"=0.0, "[56]"=0.0, "[57]"=0.0, "[58]"=0.0, "[59]"=0.0, "[60]"=0.0, "[61]"=0.0, "[62]"=0.0, "[63]"=0.0, "[64]"=0.0, "[65]"=0.0, "[66]"=0.0, "[67]"=0.0, "[68]"=0.0, "[69]"=0.0, "[71]"=0.0, "[70]"=0.0, "[0] 2"=0.0, "[1] 2"=0.0, "[2] 2"=0.0, "[3] 2"=0.0, "[4] 2"=0.0, "[5] 2"=0.0, "[6] 2"=0.0, "[7] 2"=0.0, "[8] 2"=0.0, "[9] 2"=0.0, "[10] 2"=0.0, "[11] 2"=0.0, "[12] 2"=0.0, "[13] 2"=0.0, "[14] 2"=0.0, "[15] 2"=0.0, "[16] 2"=0.0, "[17] 2"=0.0, "[18] 2"=0.0, "[19] 2"=0.0, "[20] 2"=0.0, "[21] 2"=0.0, "[22] 2"=0.0, "[23] 2"=0.0, "[24] 2"=0.0, "[25] 2"=0.0, "[26] 2"=0.0, "[27] 2"=0.0, "[28] 2"=0.0, "[29] 2"=0.0, "[30] 2"=0.0, "[31] 2"=0.0, "[32] 2"=0.0, "[33] 2"=0.0, "[34] 2"=0.0, "[35] 2"=0.0, "[36] 2"=0.0, "[37] 2"=0.0, "[38] 2"=0.0, "[39] 2"=0.0, "[40] 2"=0.0, "[41] 2"=0.0, "[42] 2"=0.0, "[43] 2"=0.0, "[44] 2"=0.0, "[45] 2"=0.0, "[46] 2"=0.0, "[47] 2"=0.0, "[48] 2"=0.0, "[49] 2"=0.0, "[50] 2"=0.0, "[51] 2"=0.0, "[52] 3"=0.0, "[53] 2"=0.0, "[54] 2"=0.0, "[55] 2"=0.0, "[56] 2"=0.0, "[57] 2"=0.0, "[58] 2"=0.0, "[59] 2"=0.0, "[60] 2"=0.0, "[61] 2"=0.0, "[62] 2"=0.0, "[63] 2"=0.0, "[64] 2"=0.0, "[65] 2"=0.0, "[66] 2"=0.0, "[67] 2"=0.0, "[68]2"=0.0, "[69]2"=0.0, "[70]2"=0.0, "[71]2"=0.0, "[0] 3"=0.0, "[1] 3"=0.0, "[2] 3"=0.0, "[3] 3"=0.0, "[4] 3"=0.0, "[5] 3"=0.0, "[6] 3"=0.0, "[7] 3"=0.0, "[8] 3"=0.0, "[9] 3"=0.0, "[10] 3"=0.0, "[11] 3"=0.0, "[12] 3"=0.0, "[13] 3"=0.0, "[14] 3"=0.0, "[15] 3"=0.0, "[16] 3"=0.0, "[17] 3"=0.0, "[18] 3"=0.0, "[19] 3"=0.0, "[20] 3"=0.0, "[21] 3"=0.0, "[22] 3"=0.0, "[23] 3"=0.0, "[24] 3"=0.0, "[25] 3"=0.0, "[26] 3"=0.0, "[27] 3"=0.0, "[28] 3"=0.0, "[29] 3"=0.0, "[30] 3"=0.0, "[31] 3"=0.0, "[32] 3"=0.0, "[33] 3"=0.0, "[34] 3"=0.0, "[35] 3"=0.0, "[36] 3"=0.0, "[37] 3"=0.0, "[38] 3"=0.0, "[39] 3"=0.0, "[40] 3"=0.0, "[41] 3"=0.0, "[42] 3"=0.0, "[43] 3"=0.0, "[44] 3"=0.0, "[45] 3"=0.0, "[46] 3"=0.0, "[47] 3"=0.0, "[48] 3"=0.0, "[49] 3"=0.0, "[50] 3"=0.0, "[51] 3"=0.0, "[52] 4"=0.0, "[53] 3"=0.0, "[54] 3"=0.0, "[55] 3"=0.0, "[56] 3"=0.0, "[57] 3"=0.0, "[58] 3"=0.0, "[59] 3"=0.0, "[60] 3"=0.0, "[61] 3"=0.0, "[62] 3"=0.0, "[63] 3"=0.0, "[64] 3"=0.0, "[65] 3"=0.0, "[66] 3"=0.0, "[67] 3"=0.0, "[68]3"=0.0, "[69]3"=0.0, "[70]3"=0.0, "[71]3"=0.0, "[4] 4"=0.0, "[5] 4"=0.0, "[6] 4"=0.0, "[7] 4"=0.0, "[8] 4"=0.0, "[9] 4"=0.0, "[10] 4"=0.0, "[11] 4"=0.0, "[12] 4"=0.0, "[13] 4"=0.0, "[14] 4"=0.0, "[15] 4"=0.0, "[16] 4"=0.0, "[17] 4"=0.0, "[18] 4"=0.0, "[19] 4"=0.0, "[20] 4"=0.0, "[21] 4"=0.0, "[22] 4"=0.0, "[23] 4"=0.0, "[24] 4"=0.0, "[25] 4"=0.0, "[26] 4"=0.0, "[27] 4"=0.0, "[28] 4"=0.0, "[29] 4"=0.0, "[30] 4"=0.0, "[31] 4"=0.0, "[32] 4"=0.0, "[33] 4"=0.0, "[17] 9"=0.0, "[0] 9"=0.0, "[51] 8"=0.0, "[34] 8"=0.0, "[17] 8"=0.0, "[0] 8"=0.0, "[34] 4"=0.0, "[35] 4"=0.0, "[36] 4"=0.0, "[37] 4"=0.0, "[38] 4"=0.0, "[39] 4"=0.0, "[40] 4"=0.0, "[41] 4"=0.0, "[42] 4"=0.0, "[43] 4"=0.0, "[44] 4"=0.0, "[45] 4"=0.0, "[46] 4"=0.0, "[47] 4"=0.0, "[48] 4"=0.0, "[49] 4"=0.0, "[50] 4"=0.0, "[34] 9"=0.0, "[51] 4"=0.0, "[52] 5"=0.0, "[53] 4"=0.0, "[54] 4"=0.0, "[55] 4"=0.0, "[56] 4"=0.0, "[57] 4"=0.0, "[58] 4"=0.0, "[59] 4"=0.0, "[60] 4"=0.0, "[61] 4"=0.0, "[62] 4"=0.0, "[63] 4"=0.0, "[64] 4"=0.0, "[65] 4"=0.0, "[66] 4"=0.0, "[67] 4"=0.0, "[51] 9"=0.0}, "TBMSMax"=0.0, "TBMSMin"=0.0, "TBMSMean"=0.0} ("BMS Telemetry"), x=w110) -> (*(type *) &x=w77:T2)
    "BMS Telemetry" <- w77
    n26 = local read "Telem Stop"() -> (w105:bool)
    n27 = Unbundle By Name(w77) -> ("VCells"=w100:T28)
    n28 = Unbundle By Name(w77) -> ("TBMSCells"=w54:T29)
    n29 = Cluster To Array(cluster=w100) -> (array=w83:dbl[])
    n30 = Build Array (concatenate)(w95, w94, w93, w92) -> (w53:i32[])
    n31 = Array Subset(array=w83, index=0, length=18) -> (w74:dbl[])
    n32 = Cluster To Array(cluster=w54) -> (array=w55:dbl[])
    n33 = Array Subset(array=w55, index=0, length=18) -> (w57:dbl[])
    n34 = Array Subset(array=w83, index=18, length=18) -> (w79:dbl[])
    n35 = Reverse 1D Array(array=w79) -> (reversed array=w75:dbl[])
    n36 = Array Subset(array=w83, index=36, length=18) -> (w73:dbl[])
    n37 = Array Subset(array=w55, index=18, length=18) -> (w61:dbl[])
    n38 = Reverse 1D Array(array=w61) -> (reversed array=w58:dbl[])
    n39 = Array Subset(array=w83, index=54, length=17) -> (w81:dbl[])
    n40 = Array Subset(array=w55, index=36, length=18) -> (w56:dbl[])
    n41 = Array Subset(array=w55, index=54, length=17) -> (w63:dbl[])
    n42 = Insert Into Array(array=w81, new element=0.0 ("new element/subarray")) -> (w78:dbl[])  [unwired: 1 in]
    n43 = Reverse 1D Array(array=w78) -> (reversed array=w76:dbl[])
    n44 = Build Array(w74, w75, w73, w76) -> (w82:dbl[][])
    n45 = call-poly <vilib>:"Plot Helper.vi"("z matrix"=w82, "y vector"=w53) -> ("3D Plot lvclass Array out"=→"Cell Voltages":refnum<class "3D Plot Datatype.lvclass">[])  [unwired: 1 in, 8 out]
    n46 = Insert Into Array(array=w63, new element=0.0 ("new element/subarray")) -> (w60:dbl[])  [unwired: 1 in]
    n47 = Reverse 1D Array(array=w60) -> (reversed array=w59:dbl[])
    n48 = Build Array(w57, w58, w56, w59) -> (w64:dbl[][])
    n49 = call-poly <vilib>:"Plot Helper.vi"("z matrix"=w64, "y vector"=w53) -> ("3D Plot lvclass Array out"=→"Cell Temps":refnum<class "3D Plot Datatype.lvclass">[])  [unwired: 1 in, 8 out]
  }
  n50 = while {
    shift-right: [w121] -> w19
    shift-left: w12 -> [w122]
    shift-right: [w119] -> w18
    shift-left: w13 -> [w123]
    stop <- "Telem Stop" stop-if-true
    n51 = UDP Read(connection ID=w123, max size (548)=2000, timeout ms (25000)=-1, 8:w122) -> (data out=w124:string, error out=w121:errorcluster, 3:w119:refnum<k16>)  [unwired: 2 out]
    n52 = Type Cast(type=T19 {"CPU Load"={"Total (%)"=0.0, "Time Critical (%)"=0.0, "Timed Structures (%)"=0.0, "High (%)"=0.0, "Above Normal (%)"=0.0, "Normal (%)"=0.0, "Background (%)"=0.0, "Idle (%)"=0.0, "ISR (%)"=0.0}, "SVehicleStatus"={"BMS Status"={"eStatusSeverity"=enum."Okay", "NValue"=0.0, "CMessage"=enum."ControllerTemperature", "bNotOK"=FALSE}, "MC Status"={"eStatusSeverity"=enum."Okay", "NValue"=0.0, "CMessage"=enum."ControllerTemperature", "bNotOK"=FALSE}, "Shutdown Status"={"eStatusSeverity"=enum."Okay", "NValue"=0.0, "CMessage"=enum."ControllerTemperature", "bNotOK"=FALSE}, "sbRIO Status"={"eStatusSeverity"=enum."Okay", "NValue"=0.0, "CMessage"=enum."ControllerTemperature", "bNotOK"=FALSE}, "Vehicle Status"={"eStatusSeverity"=enum."Okay", "NValue"=0.0, "CMessage"=enum."ControllerTemperature", "bNotOK"=FALSE}, "Shutdown State"=enum."NI.SC.Initial", "AIR Status"=enum."Off", "Remote Return to Pits"=FALSE, "Reason for Shutdown"=enum."None", "MC State Machine Status"=enum."NI.SC.Initial"}, "iPhone HF Data"={"gXiPhone"=0.0, "gYiPhone"=0.0, "gZiPhone"=0.0, "nYawXiPhone"=0.0, "nYawYiPhone"=0.0, "nYawZiPhone"=0.0}, "iPhone LF Data"={"nLatiPhone"=0.0, "nLongiPhone"=0.0, "nGPSiPhone"=0.0}, "stop"=FALSE, "VSupplyOffset"=0.0, "VsbRIOSupply"=0.0, "bFPGALED"=FALSE, "TSBRIO"=0.0, "rTPS2Unscaled"=0.0, "rTPS1Unscaled"=0.0, "bTPSConsistent"=FALSE, "bTPSInRange"=FALSE, "rThrottle"=0.0, "VTPS2"=0.0, "rTPS2"=0.0, "VTPS1"=0.0, "rTPS1"=0.0, "rTPS2Max"=0.27001953125, "rTPS2Min"=0.489990234375, "rTPS1Max"=0.6201171875, "rTPS1Min"=0.41015625, "bCoolantPumpEnable"=FALSE, "bRTDSEnable"=FALSE, "bTSMSInStatus"=FALSE, "bPosAIREnable"=FALSE, "bBMSOK"=FALSE, "bIMDOK"=FALSE, "bBSPDOK"=FALSE, "bSBRIOOK2"=FALSE, "bSBRIOOK1"=FALSE, "bTSMSOutStatus"=FALSE, "eGreenDash"=enum."Off", "eYellowDash"=enum."Off", "eRedDash"=enum."Off", "bMotorControllerEnable"=FALSE, "tCurrentLap"=0, "bNewLap"=FALSE, "tLastLap"=0, "tLapMin"=0, "V5VSupply"=0.0, "bWheelRL"=TRUE, "bWheelRR"=TRUE, "bWheelFR"=FALSE, "bWheelFL"=FALSE, "VBrakePressureR"=0.4820976257324219, "VBrakePressureF"=0.4808177947998047, "bWheelRRStopped"=FALSE, "bWheelRLStopped"=FALSE, "bWheelFRStopped"=FALSE, "bWheelFLStopped"=TRUE, "tWheelRLPeriod"=0, "tWheelRRPeriod"=0, "tWheelFRPeriod"=0, "tWheelFLPeriod"=0, "bBrakeLight"=TRUE, "VShockRR"=0.3793773651123047, "VShockRL"=0.3444976806640625, "VShockFR"=0.3425788879394531, "VShockFL"=0.3892974853515625, "IHighCurrent"=-20.724609375, "ILowCurrent"=4.353515625, "pBrakeR"=0.0, "pBrakeF"=0.0, "bHighCurrentOK"=FALSE, "bLowCurrentOK"=FALSE, "bBrakeROK"=FALSE, "bBrakeFOK"=FALSE, "VSteerWheelMiddle"=0.34827280044555664, "aSteerWheel"=124.90449142456055, "nWheelFL"=0.0, "nWheelFR"=0.0, "nWheelRL"=0.0, "nWheelRR"=0.0, "ADXL345 Output"={"X"=0.0, "Y"=0.0, "Z"=0.0}, "Tire Diameter(m)"=0.0, "vWheelRR"=0.0, "vWheelRL"=0.0, "vWheelFR"=0.0, "vWheelFL"=0.0, "vWheelLowest"=0.0, "vWheelHighest"=0.0, "bAccel"=FALSE, "vAxleF"=0.0, "vCar"=0.0, "sLap"=0.0, "rSlipRL"=0.0, "rSlipRR"=0.0, "rSlipFL"=0.0, "rSlipFR"=0.0, "NLap"=0, "tLapReference"=0, "tFastestLap"=0, "MTorqueRequest"=0.0, "RS232 Error Out"={"status"=FALSE, "code"=0}} ("Telemetry"), x=w124) -> (*(type *) &x=→"Telemetry":T19)
  }
  n53 = while {
    shift-right: [w132] -> w17
    shift-left: w21 -> [w133]
    shift-right: [w130] -> w16
    shift-left: w15 -> [w129]
    stop <- w131 stop-if-true
    n54 = UDP Read(connection ID=w133, timeout ms (25000)=-1, 8:w129) -> (data out=w134:string, error out=w130:errorcluster, 3:w132:refnum<k16>)  [unwired: 1 in, 2 out]
    n55 = Type Cast(type=T3 {"MC Temp 1"={"TMCModuleA"=0.0, "TMCModuleB"=0.0, "TMCModuleC"=0.0, "TMCGateDriver"=0.0}, "MC Temp 2"={"TMCControlBoard"=0.0, "TMCRTD1"=0.0, "TMCRTD2"=0.0, "TMCRTD3"=0.0}, "MC Temp 3"={"TMCRTD4"=0.0, "TMCRTD5"=0.0, "TMotor"=0.0, "MTorqueShudder"=0.0}, "MC Current"={"IMCPhaseA"=0.0, "IMCPhaseB"=0.0, "IMCPhaseC"=0.0, "IMCBatteryCalc"=0.0}, "MC Voltage"={"VMCPhaseAB"=0.0, "VMCPhaseBC"=0.0, "VMCOutput"=0.0, "VMCBattery"=0.0}, "MC State"={"eMCInverterState"=enum."Power On", "eMCInverterRunMode"=enum."Torque Mode", "eMCInverterCommandMode"=enum."CAN Mode", "bMCInverterEnable"=FALSE, "bMCInverterEnableLockout"=FALSE, "bMCDirectionForward"=FALSE, "eMCVSMState"=enum."VSM Start", "bMCRelay1"=FALSE, "bMCRelay2"=FALSE, "bMCRelay3"=FALSE, "bMCRelay4"=FALSE}, "MC Torque"={"MMCRequested"=0.0, "MMCFeedback"=0.0, "tMCElapsed"=0}, "MC Position"={"aMotor"=0.0, "nMotor"=0.0, "fMCOutput"=0.0, "aDeltaResolverFilt"=0.0}, "MC Faults"={"MC Fault"={"Over-Speed"=FALSE, "Over-Current"=FALSE, "Over-Voltage"=FALSE, "Inverter Over-Temp"=FALSE, "Direction Command"=FALSE, "Inverter Response Time-Out"=FALSE, "Desat Fault"=FALSE, "Hardware Over-Current"=FALSE, "Under-Voltage"=FALSE, "CAN Command Message Lost"=FALSE, "Motor Over-Temp"=FALSE, "Module A Over-Temp"=FALSE, "Module B Over-Temp"=FALSE, "Module C Over-Temp"=FALSE, "PCB Over-Temp"=FALSE, "Gate Driver 1 Over-Temp"=FALSE, "Gate Driver 2 Over-Temp"=FALSE, "Gate Drive 3 Over-Temp"=FALSE, "Current Sensor Fault"=FALSE, "Resolver Not Connected"=FALSE}, "MC Post"=0, "MC RUN"=0}, "MC Flux"={"IMCFluxCommand"=0.0, "IMCFluxFeedback"=0.0, "IMC_Id"=0.0, "IMC_Iq"=0.0}, "MC Internal Voltages"={"VMCRef1_5"=0.0, "VMCRef2_5"=0.0, "VMCRef5"=0.0, "VMCRef12"=0.0}, "Mod Index & Flux Weakening"={"NMCModulationIndex"=0.0, "IMCFluxWeakeningOutput"=0.0, "IMCIdCommand"=0.0, "IMCIqCommand"=0.0}} ("MC Telemetry"), x=w134) -> (*(type *) &x=w127:T3)
    "MC Telemetry" <- w127
    n56 = local read "Telem Stop"() -> (w131:bool)
    n57 = Unbundle By Name(w127) -> ("MC Voltage.VMCBattery"=→"Waveform Chart":dbl)
  }
  n58 = UDP Close(connection ID=w17, 8:w16) -> ()  [unwired: 2 out]
  n59 = UDP Close(connection ID=w18, 8:w19) -> ()  [unwired: 2 out]
  n60 = UDP Close(connection ID=w10, 8:w11) -> ()  [unwired: 2 out]
  n61 = UDP Close(connection ID=w2, 8:w3) -> ()  [unwired: 2 out]
